vi "MainPr(Calculation)-41.vi"() -> ()   [LabVIEW 2017]
doc: "Main Program for Tracking\nThis VI Represents Front Panel and Control Buttons for Perform Tracking\nPlease, optimize the front panel for your own monitor resolution and needs"
uses:
  <vilib>/vision/Avi.llb/IMAQ AVI2 Refnum.ctl
  <vilib>/vision/NI_Vision_Development_Module.lvlib
  <vilib>/Utility/config.llb/NI_LVConfig.lvlib
panel:
  out "error out":errorcluster
  in  "STOP Program":bool
  in  "Front Panel":T1(tab)
  in  "FrameCtl":u32 max=299
  out "1st Movie (Comparison)":T2(plugin-control)
  out "1st Movie":T2(plugin-control)
  in  "Gamma":sgl format="%.2f"
  in  "Operator G Correction":T3(ring)
  in  "Parameter LoG":sgl format="%.2f"
  in  "Operator LoG":T3(ring)
  in  "1/2 Channels":bool
  in  "Sigma":dbl min=0.1
  in  "FrameCtl2":u32 max=299
  in  "Gray or Binarized?":bool
  out "1st Movie Original":T2(plugin-control)
  out "1st Movie Processed":T2(plugin-control)
  in  "Index for thresholding":i8 min=-4
  in  "Keep Nega-\ntive Values?":bool
  out "Detection Progress":u8(slide) scale=0.0..100.0
  in  "# of Frame":u32 max=299
  in  "Save pics (ex)":bool
  in  "Find ALL objects":bool
  out "Results on 1st Movie":T2(plugin-control)
  out "1st Filtering":T2(plugin-control)
  in  "Try my filters!":bool
  in  "# Erosion":i32=2
  in  "Connectivity":bool=TRUE
  in  "Min  Diam":dbl
  in  "Max  Diam":dbl min=12.0
  in  "Filter Tracks":bool
  out "Tracking progress":u8(slide) scale=0.0..100.0
  in  "Save pictures":bool
  in  "Save movies":bool
  in  "Frame":u32 max=299
  in  "Delete Tracs":bool
  out "1st Filtered":T2(plugin-control)
  in  "dR max":dbl min=1.0
  out "1st Filtering (NN)":T2(plugin-control)
  in  "dR min":dbl min=0.0 max=11.0
  out "Raw #":i32
  out "Saved #":i32
  in  "Tracking Procedure":bool
  in  "Min TRK L":i32 min=2 max=298 step=1
  in  "Closing gaps":i32 min=1 max=298 step=1
  in  "% linearity":i32 min=1 max=100 step=1
  in  "Max angle":dbl min=0.0 max=89.0 step=1.0
  in  "FPS":u32
  in  "FPS Gr":u32
  in  "Save videos \nbelow as *avi":bool
  in  "Save pics below":bool
  in  "Testing Frame":u32 max=17
  out "After Resolving Correspondence Problem":T2(plugin-control)
  out "Connected and Grouped Tracks":T2(plugin-control)
  in  "Tracks group":i32 min=0 max=394
  in  "Save Tracks in Columns (x,y,dx,dy)":bool
  in  "Save Duration of Tracks":bool
  in  "Save Mean Velocities":bool
  out "Duration of Tracks":T4(graph)
  out "Mean Instant Velocities for Each Track":T4(graph)
  in  "Show Distributions":bool
  out "All Path Vels":T4(graph)
  out "All Instant Vels":T4(graph)
  out "mean Instant Vel":dbl format="%#_1f"
  out "StD Instant":dbl format="%#_1g"
  out "mean Path Vel":dbl format="%.1f"
  out "StD Path":dbl format="%.1f"
  in  "Bins":i32=10
  in  "Save All Instant Vels":bool
  in  "Save Path Velocities":bool
  # "Two channels"
  # "*Planning develop-\nment switcher (old)"
  # "One channel"
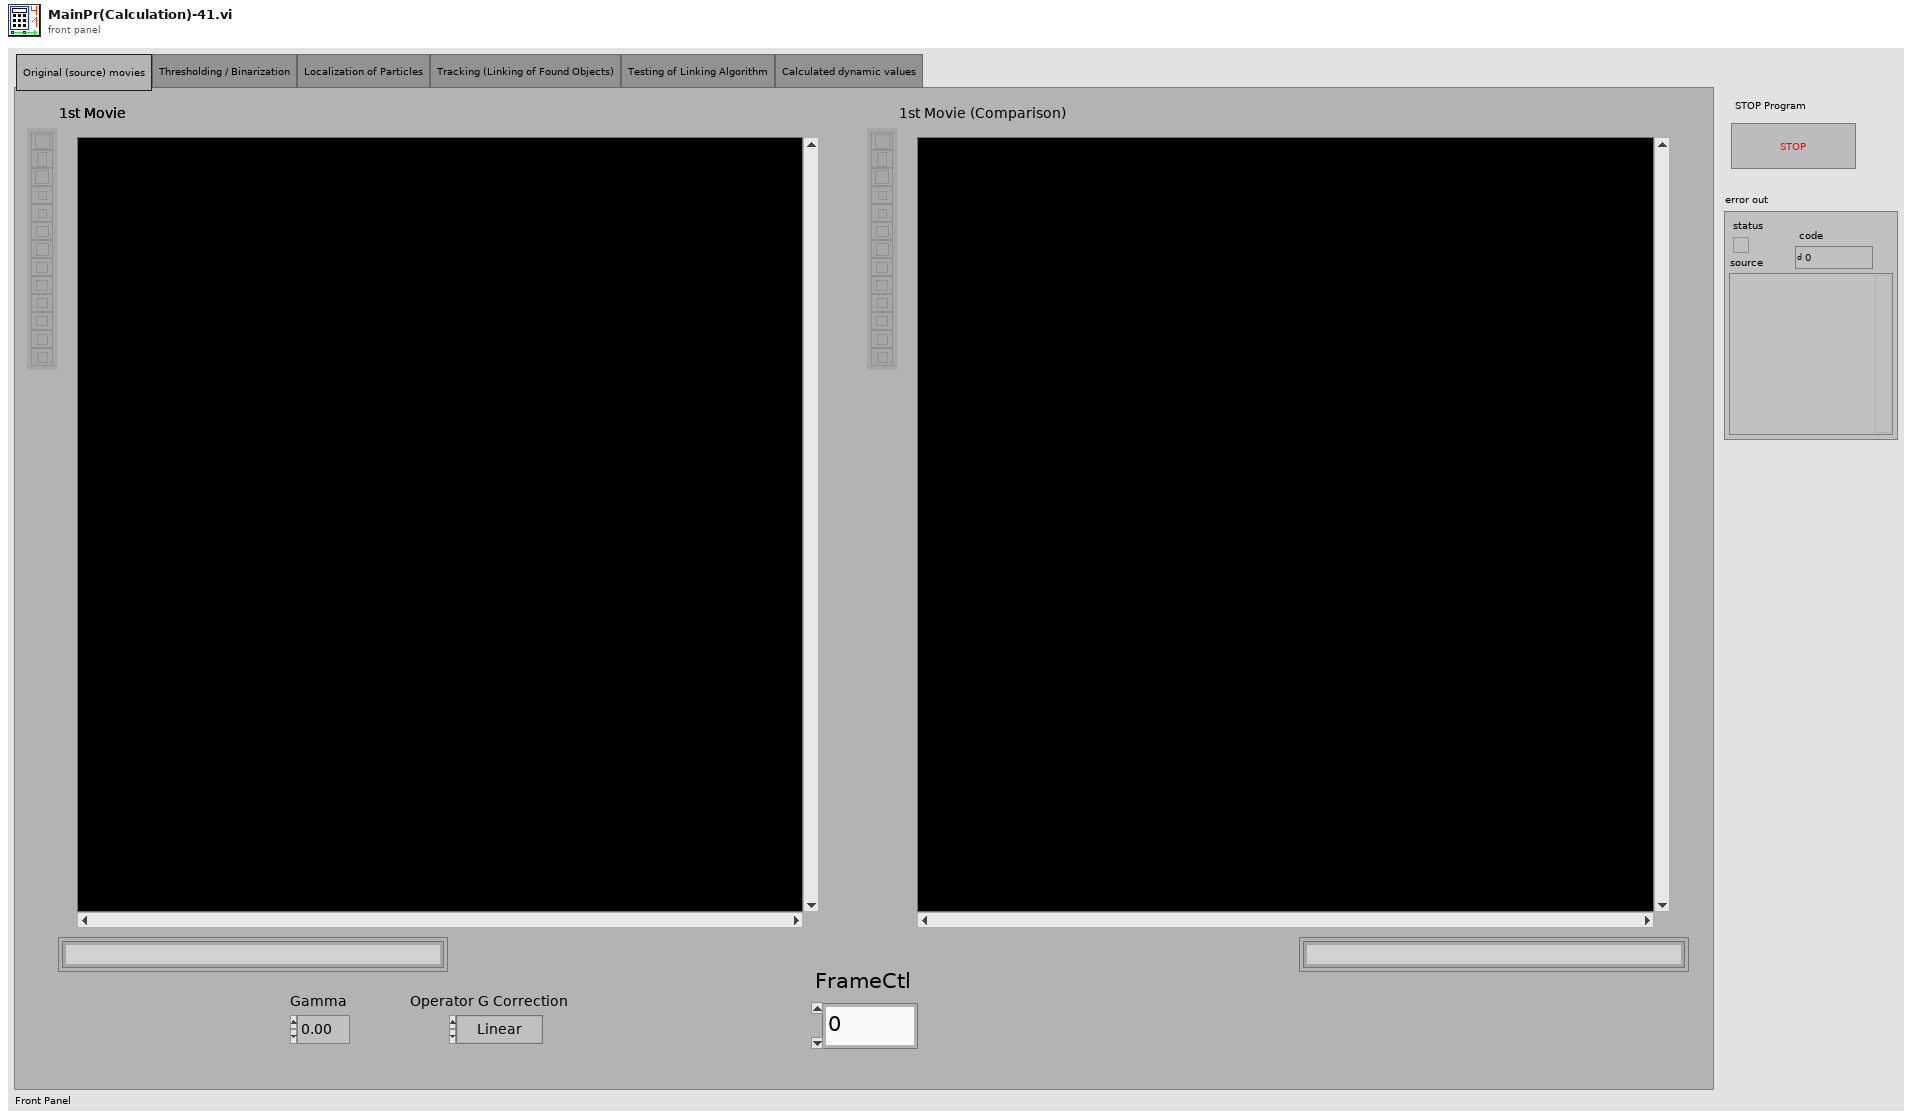
[diagram p1: front panel]
types:
  T1 = enum32{"Original (source) movies", "Thresholding / Binarization", "Localization of Particles", "Tracking (Linking of Found Objects)", "Testing of Linking Algorithm", "Calculated dynamic values"}
  T2 = typedef "IMAQ Image.ctl" = refnum<image>
  T3 = enum32{"Linear", "Log", "Exp", "Square", "Square root", "Power X", "Power 1/X"}
  T4 = cluster{"X Values":dbl[], "Histogram: h(x)":i32[]}
  T5 = typedef "IMAQ AVI2 Refnum.ctl" = refnum<k20>
  T6 = typedef "Image Type" = u32
  T7 = typedef "Particle Parameters" = i32
  T8 = cluster{"[IN] AVI Refnum":T5, "[IN] Image Type":T6, "[IN] Particle Filter Setups":cluster{"Erosion":i32, "Connectivity ":bool, "Type of particle filter":cluster{"Measurement Parameter":T7, "Min  Diam":dbl, "Max  Diam":dbl, "Range":bool, "Range":bool}[]}, "[IN] # Channel":u8, "[IN] Keep Nega-\ntive Values?":bool, "[IN] Image Filtering Settings":cluster{"Gamma Origin":sgl, "Operator Origin":enum32{"Linear", "Log", "Exp", "Square", "Square root", "Power X", "Power 1/X"}, "Gamma LoG":sgl, "Operator LoG":enum32{"Linear", "Log", "Exp", "Square", "Square root", "Power X", "Power 1/X"}, "Sigma":dbl, "Thresholding Index":i8}, "[IN] Binarization Settings":cluster{"MinBin2":sgl, "MaxBin2":sgl}[]}
  T9 = enum8{"Enabled", "Disabled", "Disabled and Grayed Out"}
  T10 = cluster{"dR min ":dbl, "dR max ":dbl, "Closing gaps":i32, "Min TRK L":i32, "% linearity":i32, "Max angle":dbl, "Tracking progress":refnum<vi>}
  T11 = typedef "NI_LVConfig.lvlib/Config Data RefNum.ctl" = refnum<k1>
  T12 = cluster{"X,Y":dbl[][], "Areas particles":dbl[][], "Particle Fil Setups":cluster{"Erosion":i32, "Connectivity ":bool, "Type of particle filter":cluster{"Measurement Parameter":T7, "Min  Diam":dbl, "Max  Diam":dbl, "Range":bool, "Range":bool}[]}, "Tracks, Coordinates":cluster{"(X,Y) Unmoved":dbl[][], "(X,Y,dX,dY) Dur 1 Frame":dbl[][], "(X,Y,dX,dY) W/t Problems":dbl[][], "(X,Y,dX,dY) NN filtered":dbl[][], "(X,Y,dX,dY) TH filtered":dbl[][], "Tracks":cluster{"Tracks":dbl[], "Start Pos":i32}[], "Tracks w/t Problems":cluster{"Tracks":dbl[], "Start Pos":i32}[]}}
  T13 = cluster{"Before Grouped Tracks":cluster{"Tracks":dbl[][], "Start Pos":i32[], "Dot Statuses":i16[][]}[], "After Grouped Tracks":cluster{"Tracks":dbl[][], "Start Pos":i32[], "Dot Statuses":i16[][]}[], "Current\nGroup":i32}
  T14 = cluster{"Gamma Origin":sgl, "Operator Origin":enum32{"Linear", "Log", "Exp", "Square", "Square root", "Power X", "Power 1/X"}, "Gamma LoG":sgl, "Operator LoG":enum32{"Linear", "Log", "Exp", "Square", "Square root", "Power X", "Power 1/X"}, "Sigma":dbl, "Thresholding Index":i8}
  T15 = cluster{"Instant Velocities (All)":dbl[], "Path Velocities (All) ":dbl[], "Tracks in columns":dbl[][], "Mean Instant Velo\ncities for Tracks":dbl[], "MSD":dbl[], "Track duration in frames":u16[], "Track length in pixels":dbl[]}
  T16 = cluster{"Starting Value":sgl, "Incremental Value":sgl, "Histogram":u32[]}
  T17 = cluster{"Erosion":i32, "Connectivity ":bool, "Type of particle filter":cluster{"Measurement Parameter":T7, "Min  Diam":dbl, "Max  Diam":dbl, "Range":bool, "Range":bool}[]}
  T18 = cluster{"Measurement Parameter":T7, "Min  Diam":dbl, "Max  Diam":dbl, "Range":bool, "Range":bool}[]
  T19 = cluster{"Tracks W/T Problems":dbl[], "Start Pos":i32}[]
  T20 = cluster{"All Instant Vel-s":cluster{"X Values":dbl[], "Histogram: h(x)":i32[]}, "mean":dbl, "standard deviation":dbl, "All Path Vel-s":cluster{"X Values":dbl[], "Histogram: h(x)":i32[]}, "mean":dbl, "standard deviation":dbl, "Mean Instan Vel-s":cluster{"X Values":dbl[], "Histogram: h(x)":i32[]}, "mean":dbl, "standard deviation":dbl, "Duration of tracks":cluster{"X Values":dbl[], "Histogram: h(x)":i32[]}, "mean":dbl, "standard deviation":dbl}
  T21 = cluster{"(X,Y) Unmoved":dbl[][], "(X,Y,dX,dY) Dur 1 Frame":dbl[][], "(X,Y,dX,dY) W/t Problems":dbl[][], "(X,Y,dX,dY) NN filtered":dbl[][], "(X,Y,dX,dY) TH filtered":dbl[][], "Tracks":cluster{"Tracks":dbl[], "Start Pos":i32}[], "Tracks w/t Problems":cluster{"Tracks":dbl[], "Start Pos":i32}[]}
  T22 = cluster{"Tracks":dbl[][], "Start Pos":i32[], "Dot Statuses":i16[][]}[]
  T23 = cluster{"[IN] Grouped Tracks":cluster{"Tracks":dbl[][], "Start Pos":i32[], "Dot Statuses":i16[][]}[], "[IN] Tracks group":i32, "[IN] Testing Frame ":u32}
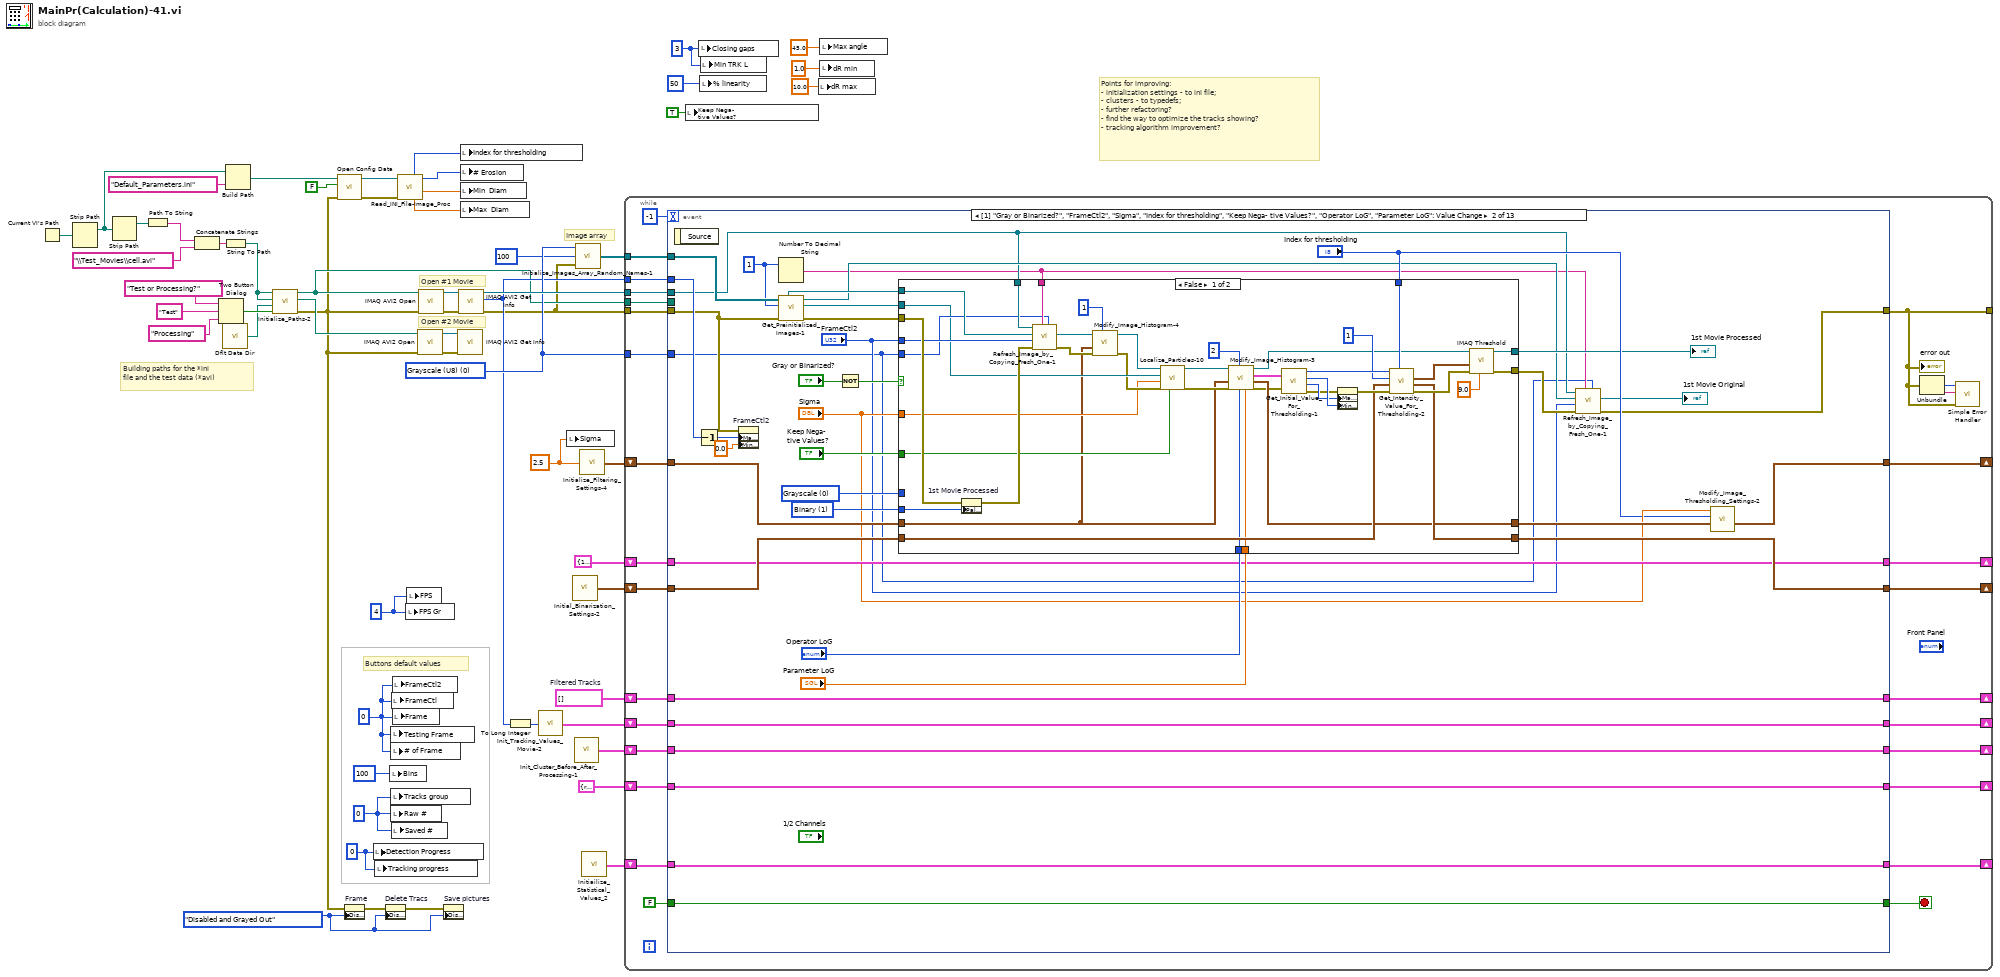
[diagram p0: block diagram]
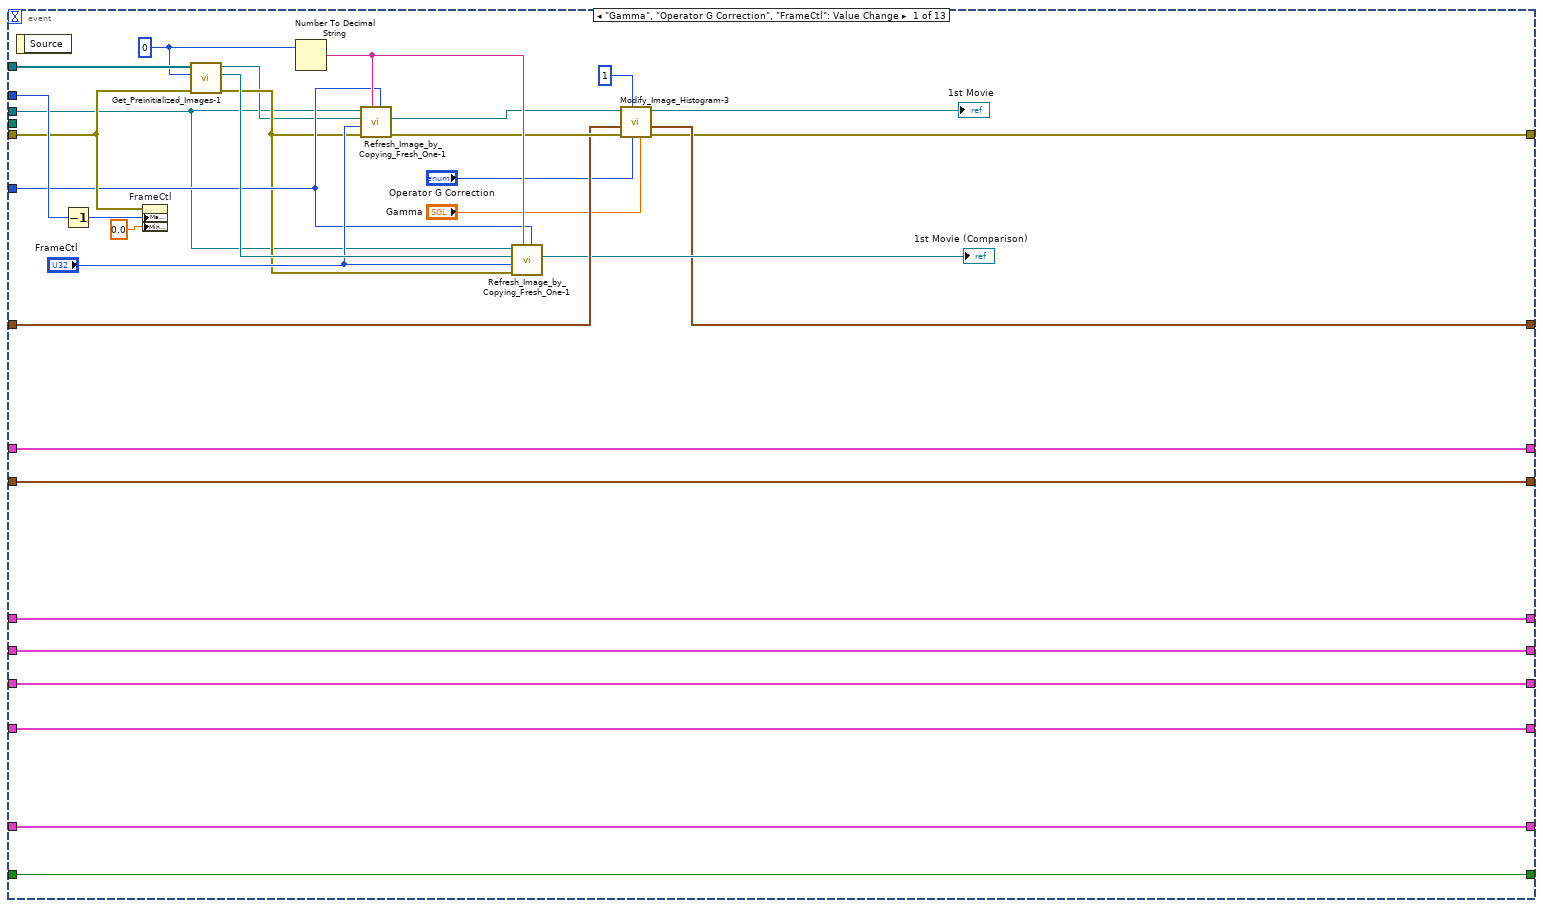
[diagram p2: hidden frame]
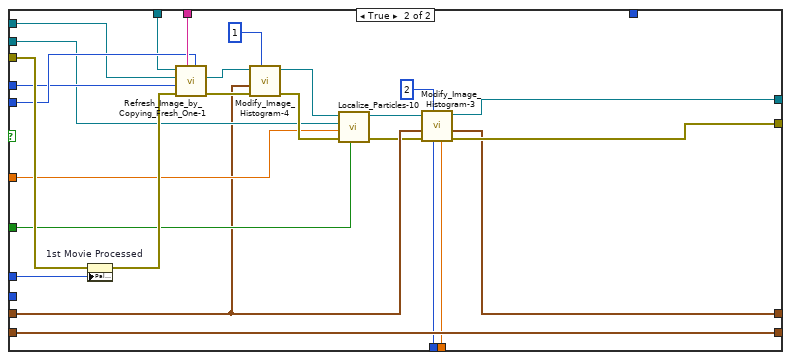
[diagram p3: hidden frame]
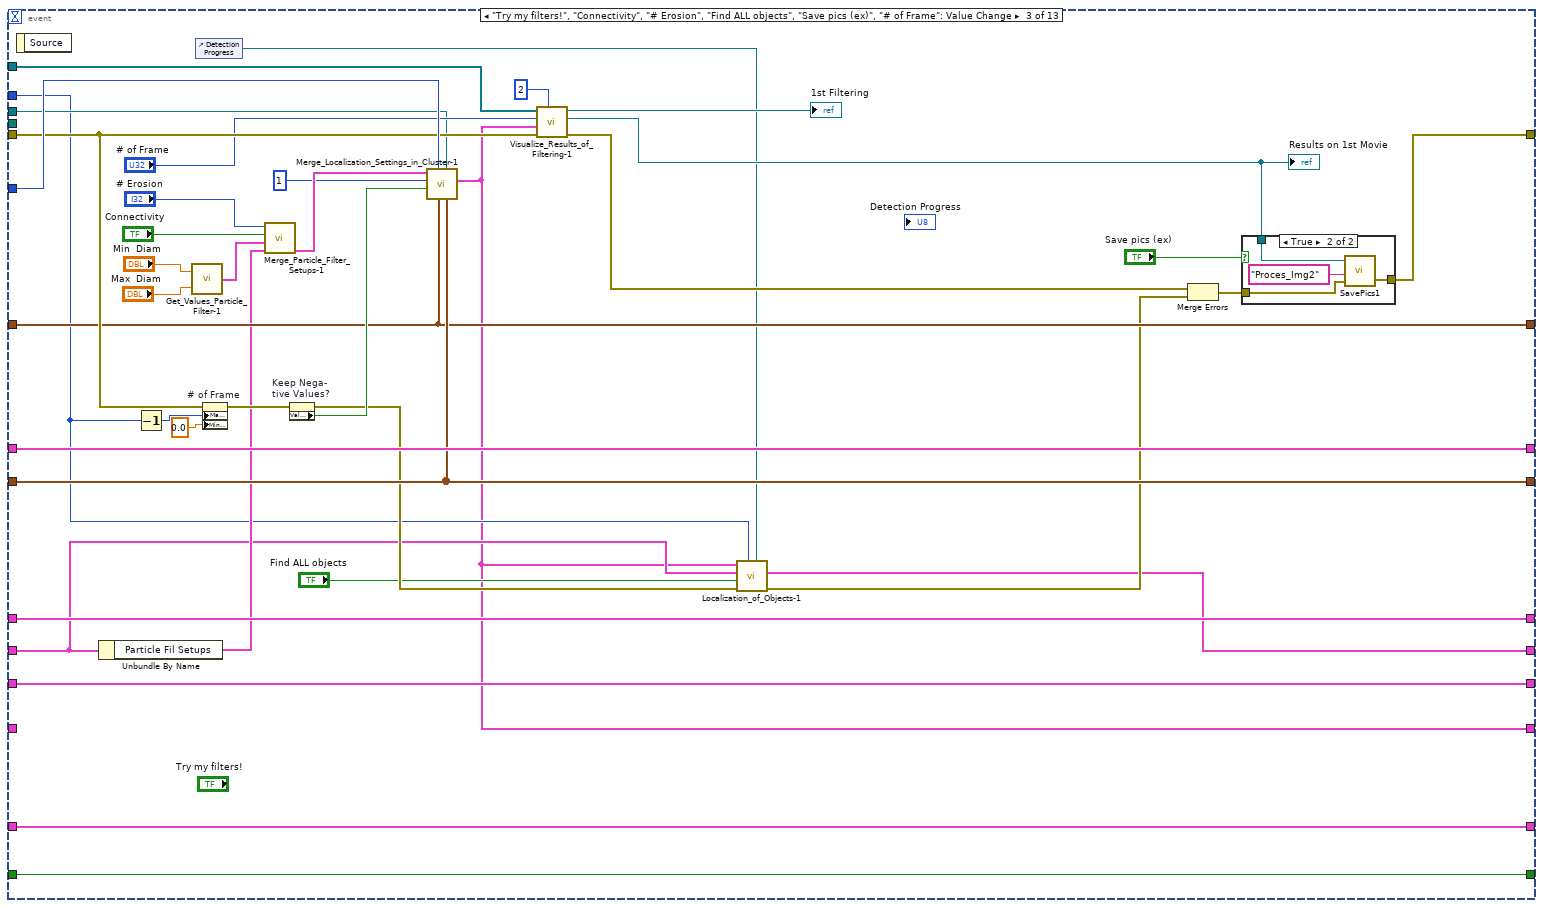
[diagram p4: hidden frame]
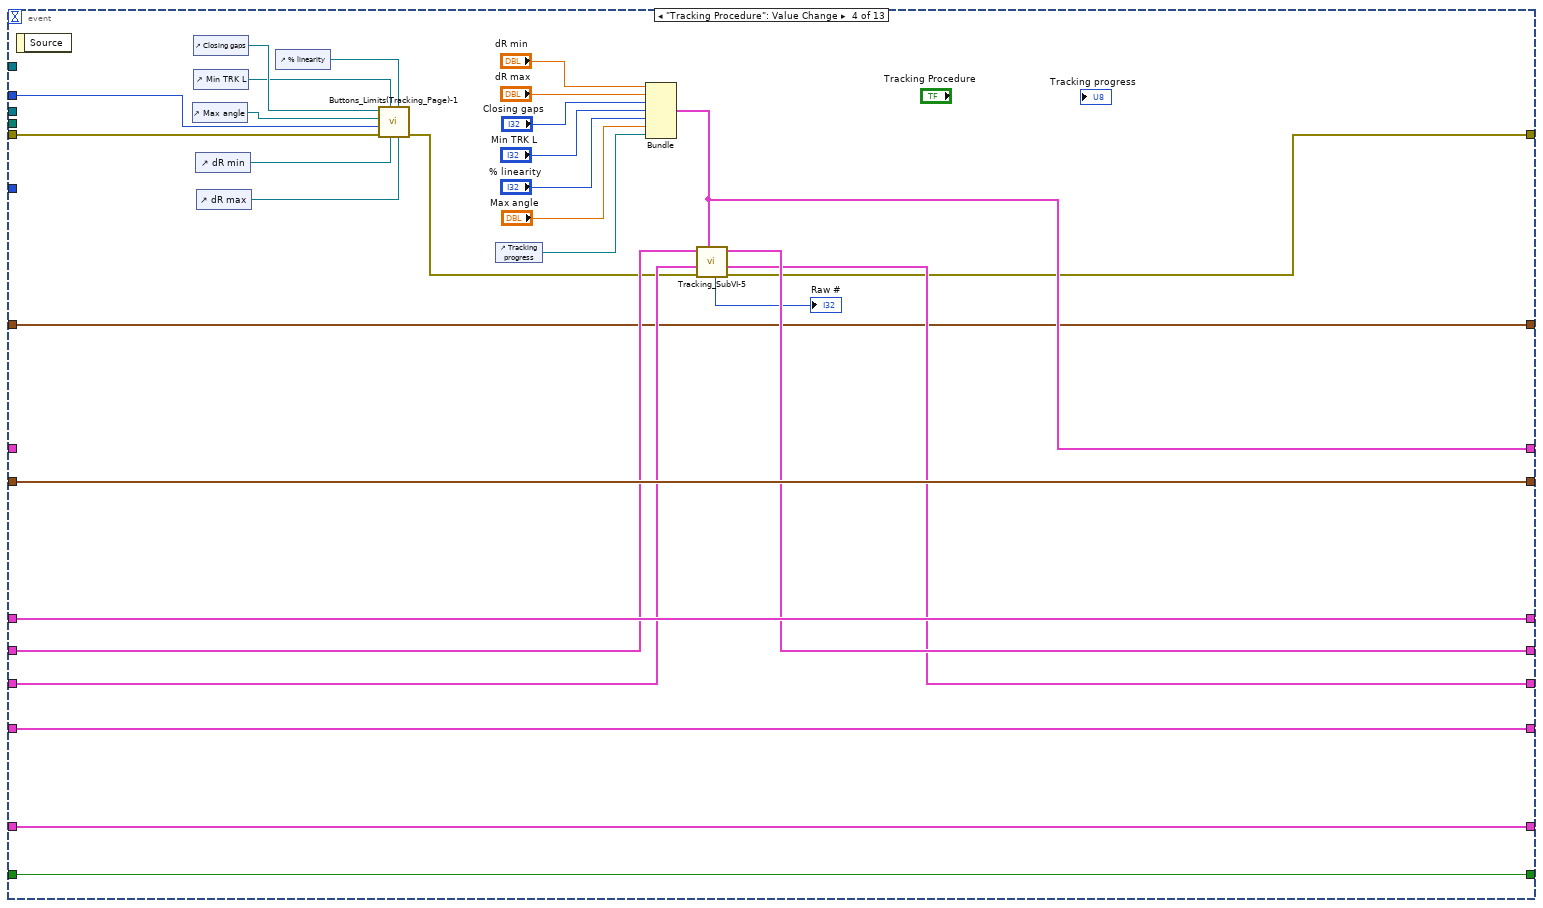
[diagram p6: hidden frame]
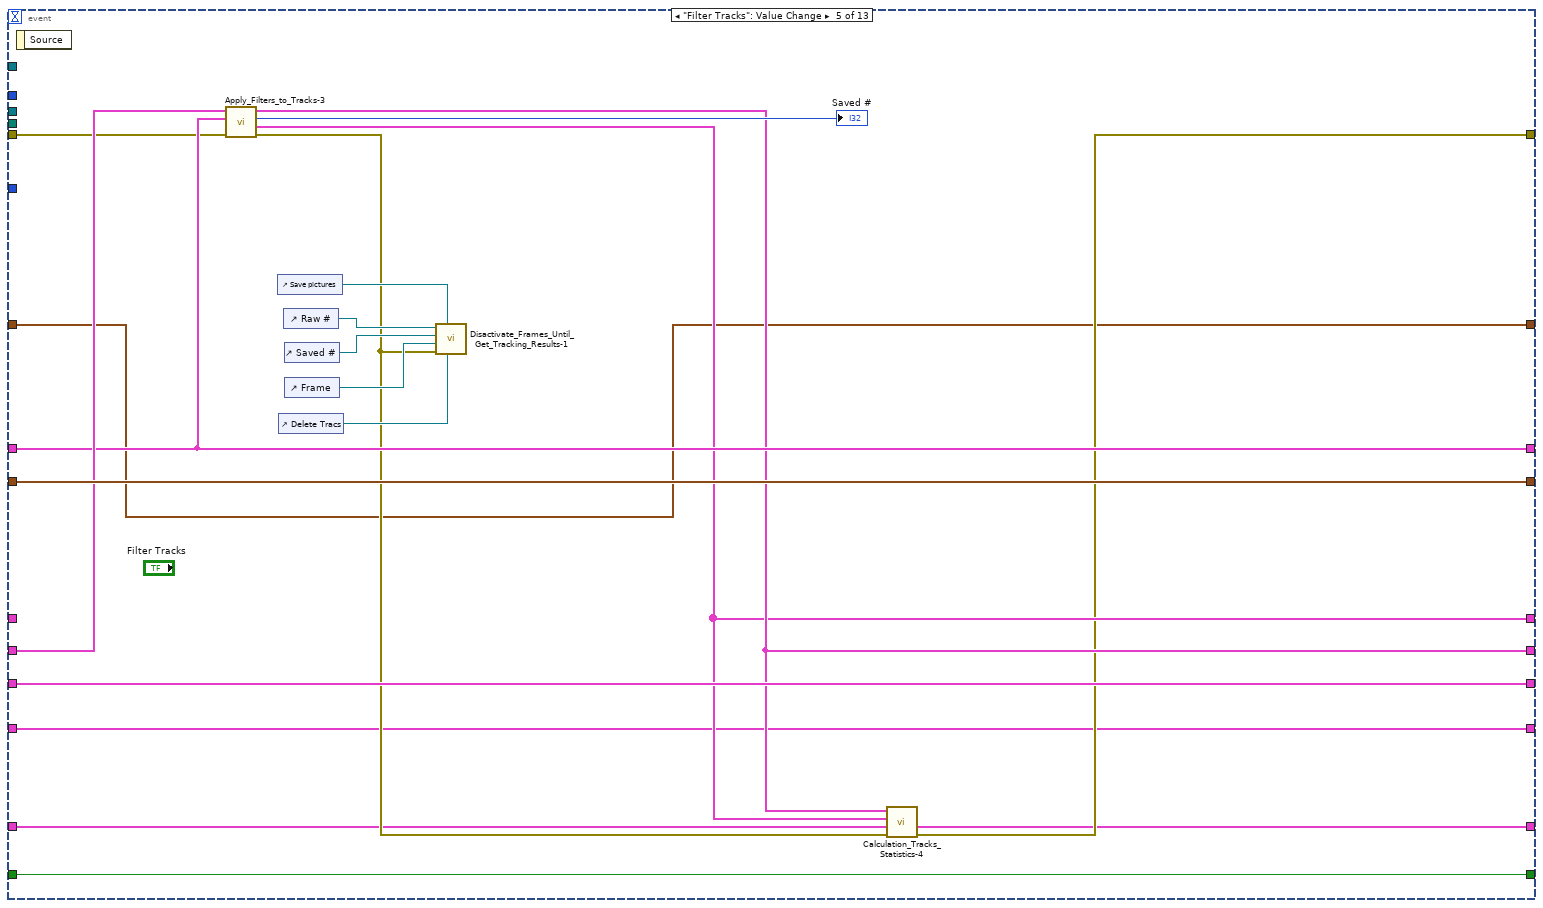
[diagram p7: hidden frame]
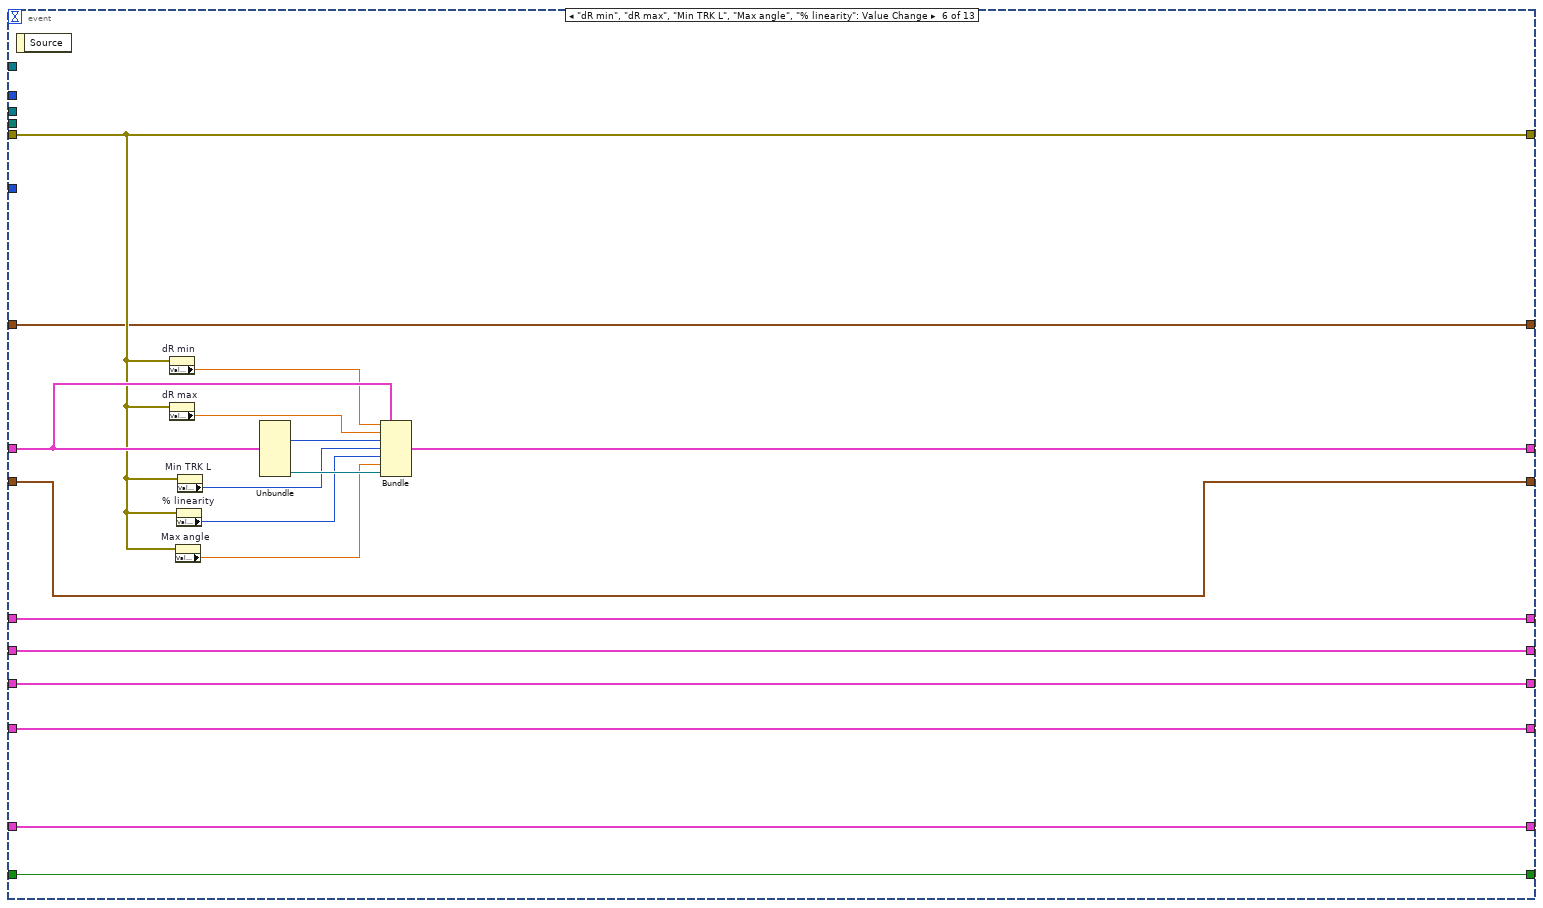
[diagram p8: hidden frame]
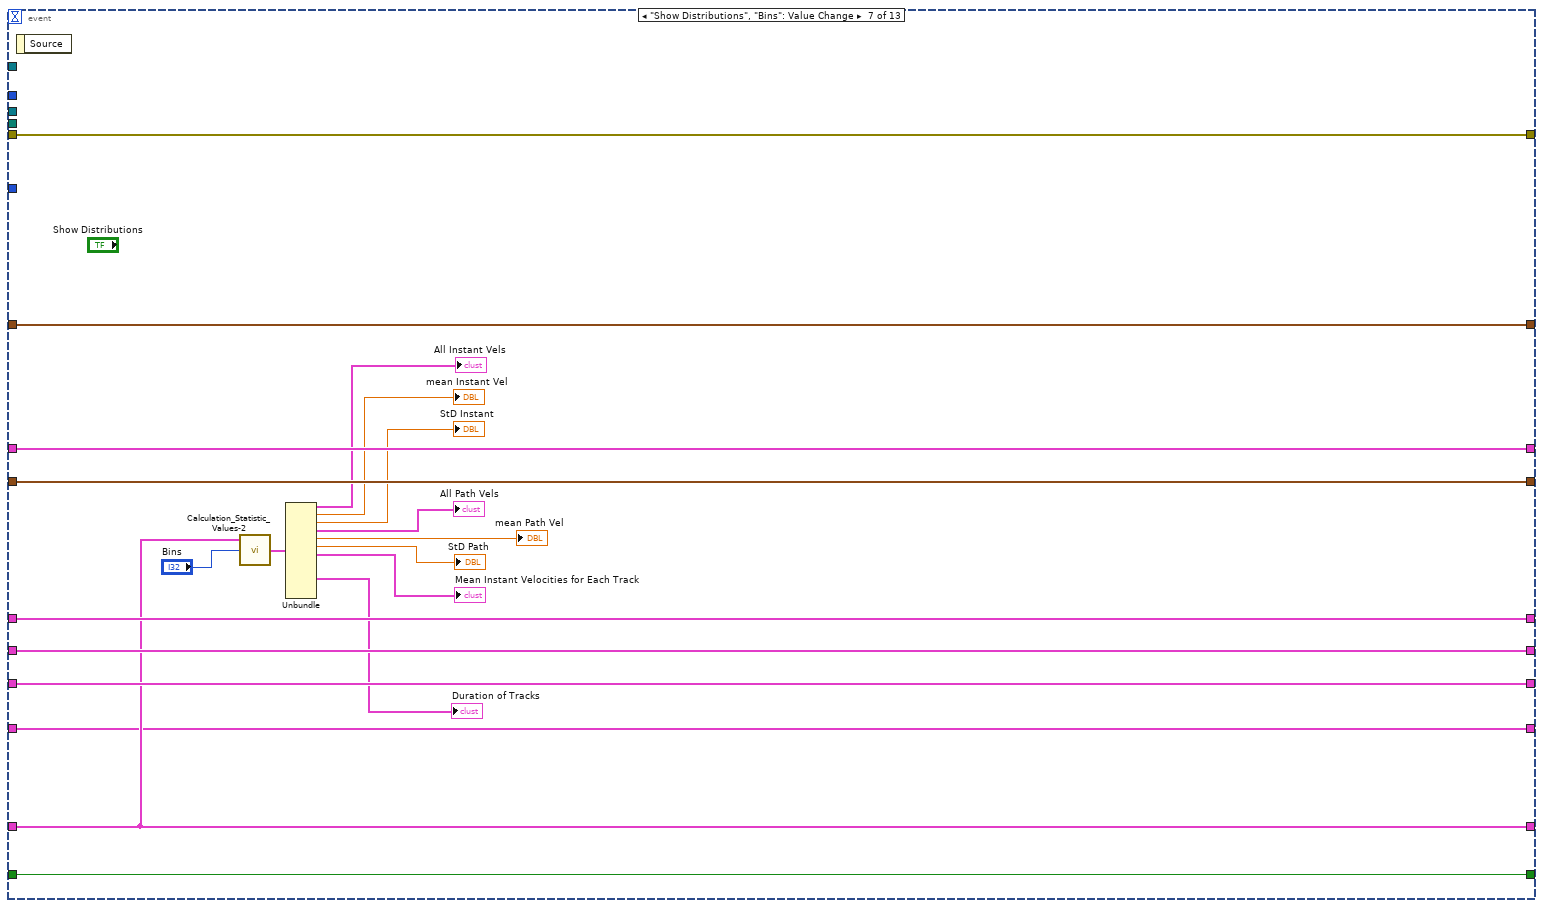
[diagram p9: hidden frame]
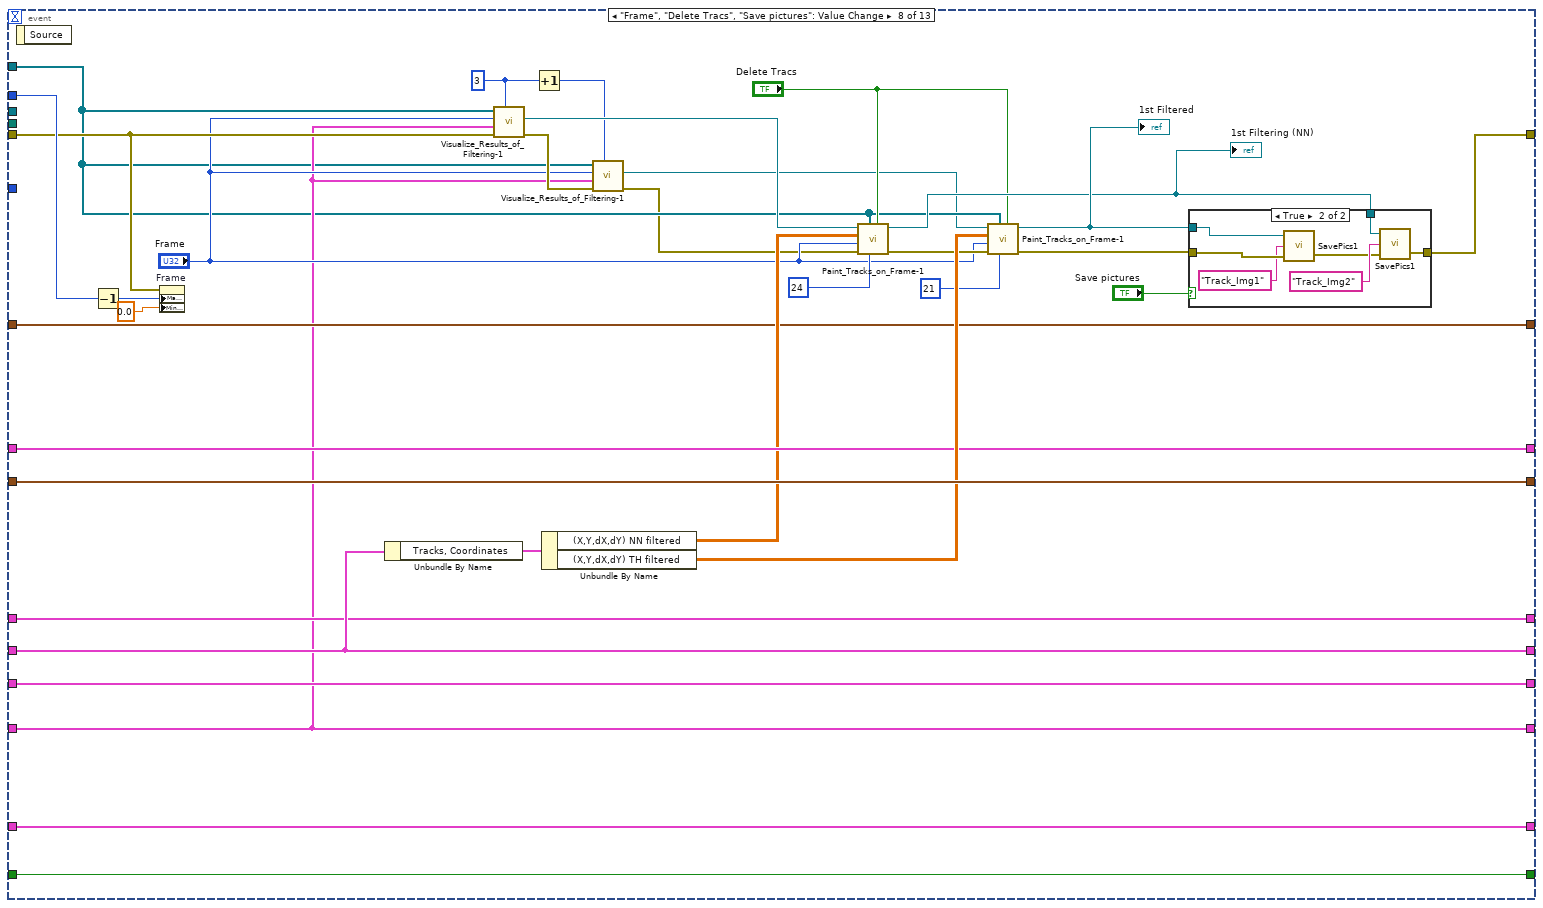
[diagram p10: hidden frame]
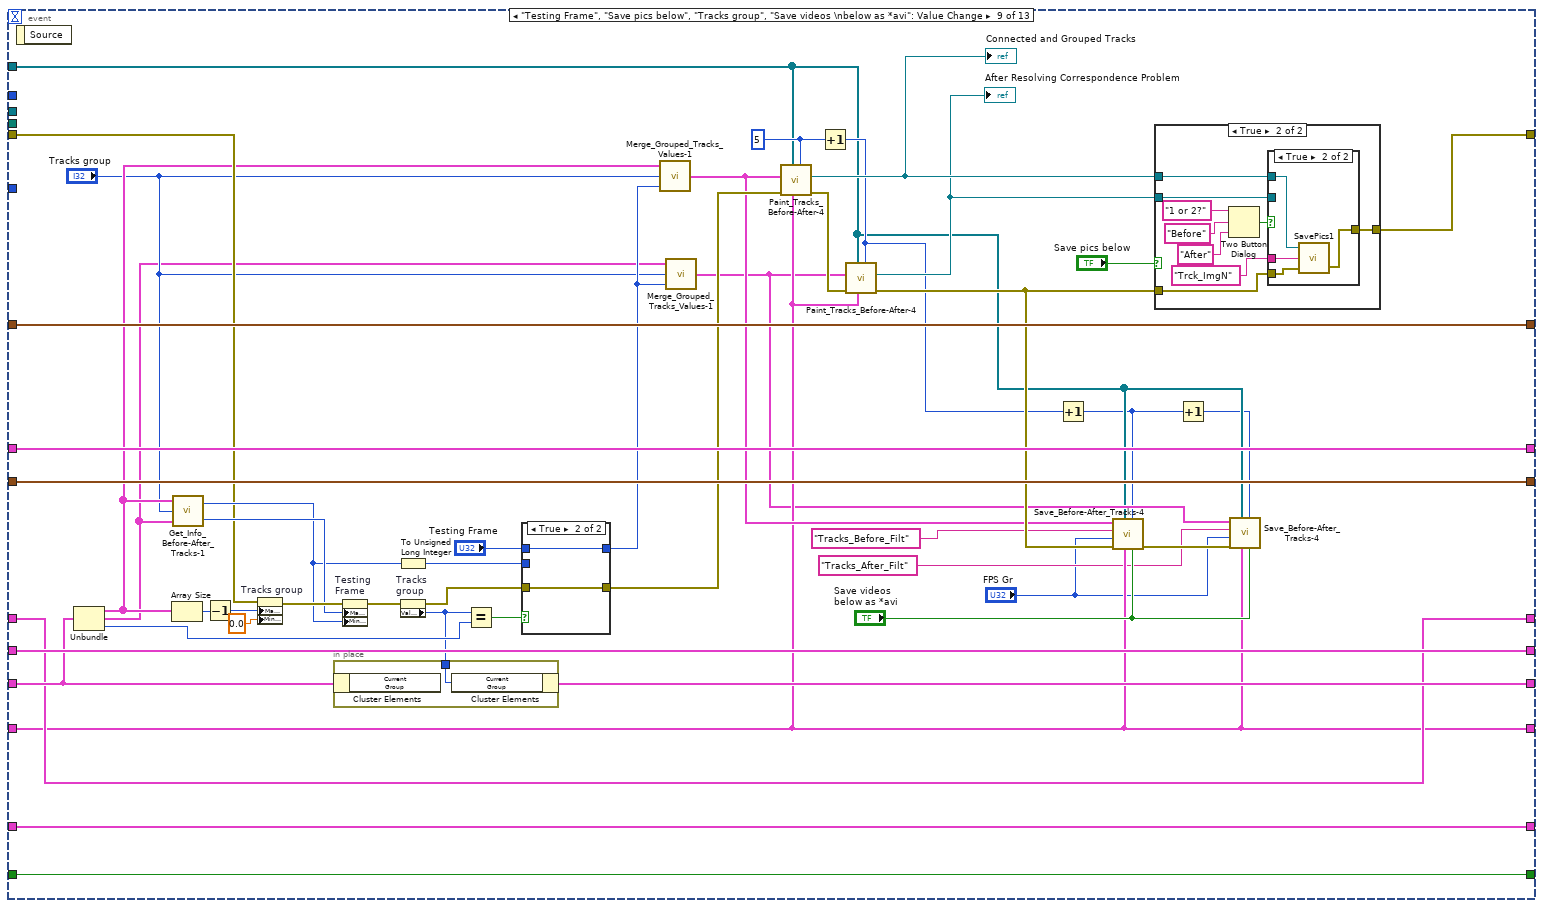
[diagram p12: hidden frame]
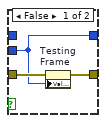
[diagram p13: hidden frame]
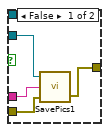
[diagram p15: hidden frame]
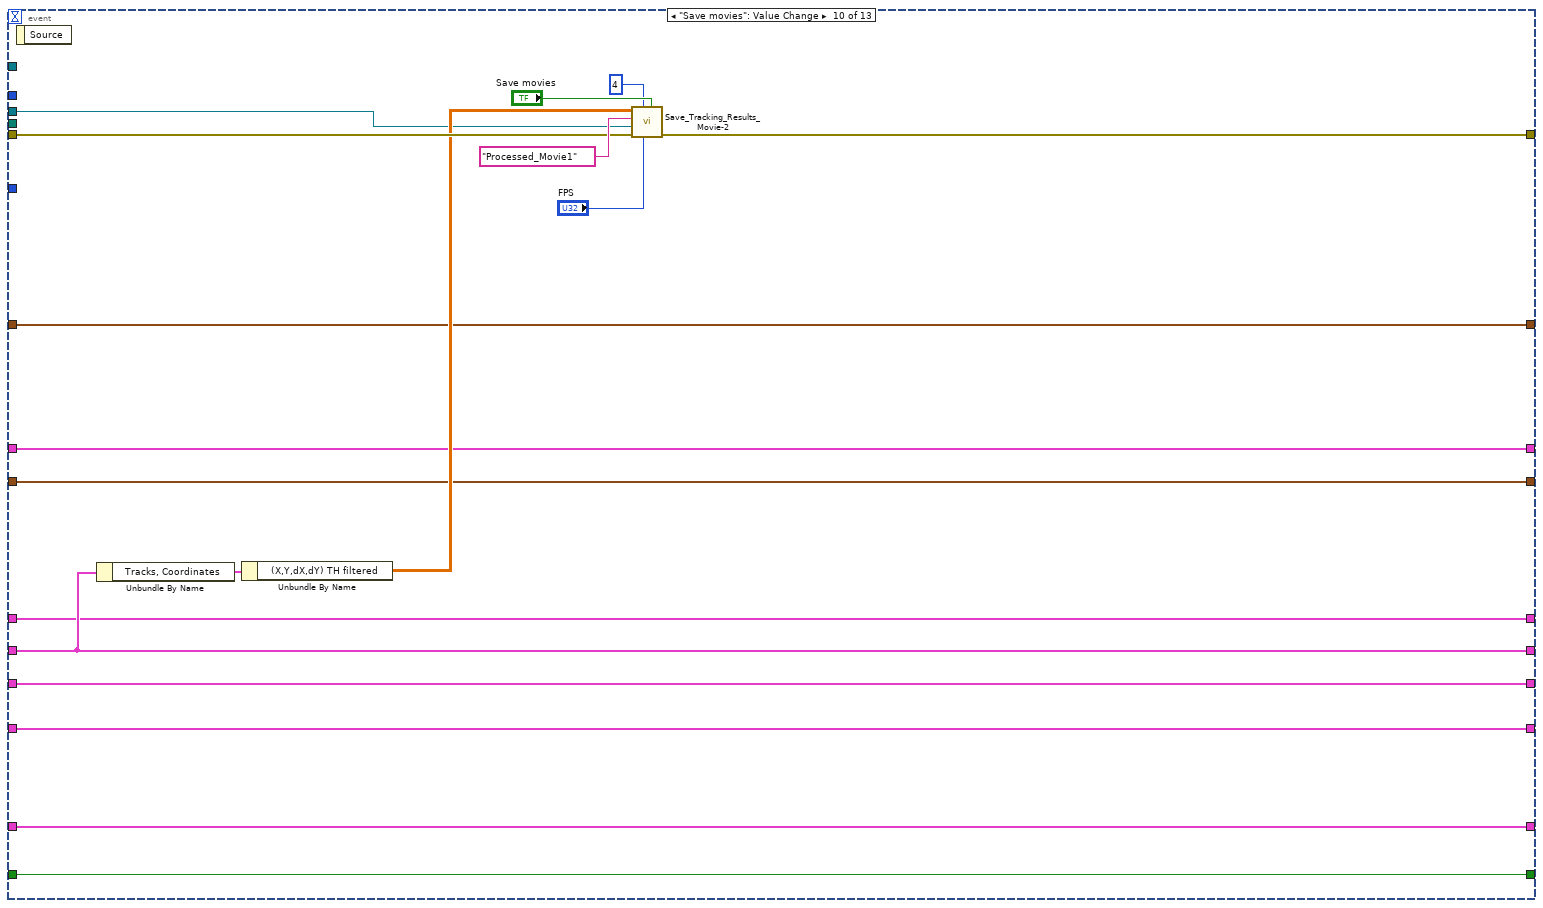
[diagram p16: hidden frame]
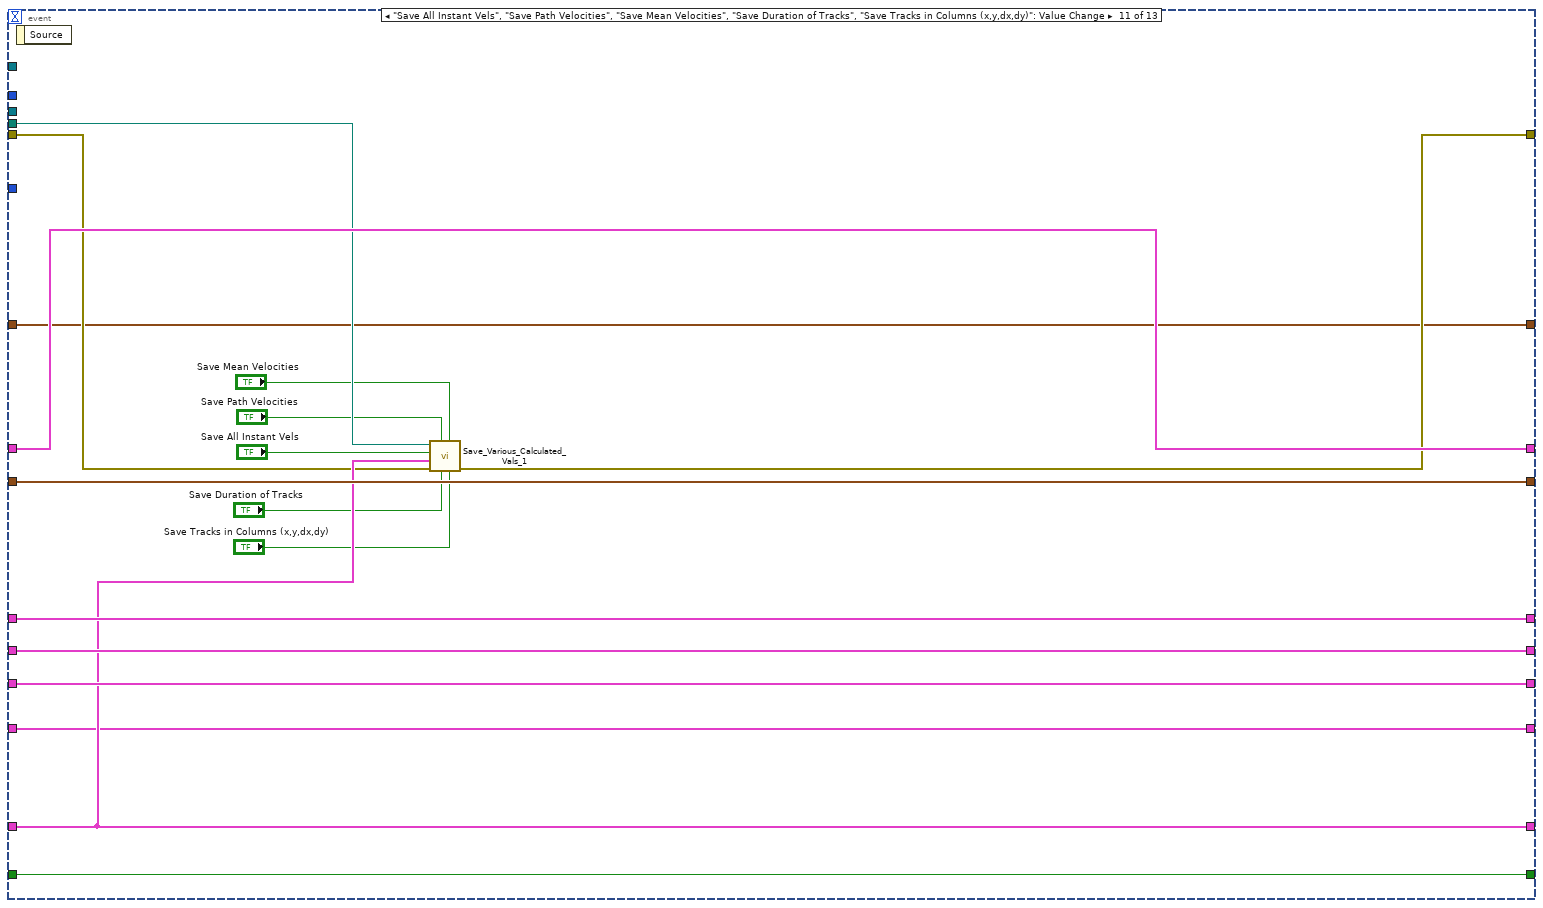
[diagram p17: hidden frame]
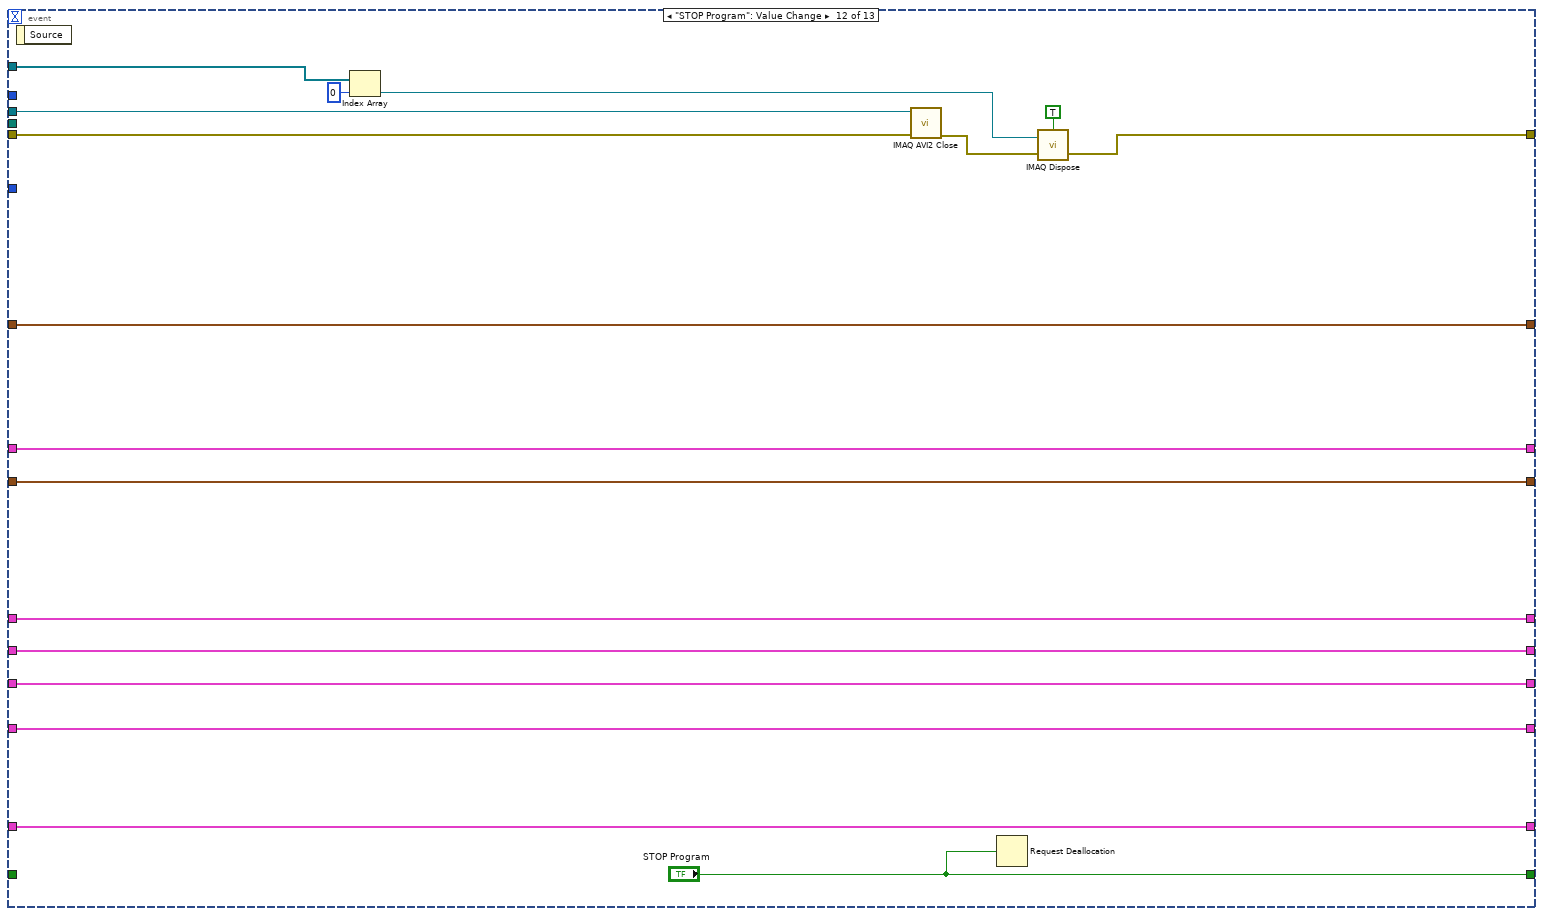
[diagram p18: hidden frame]
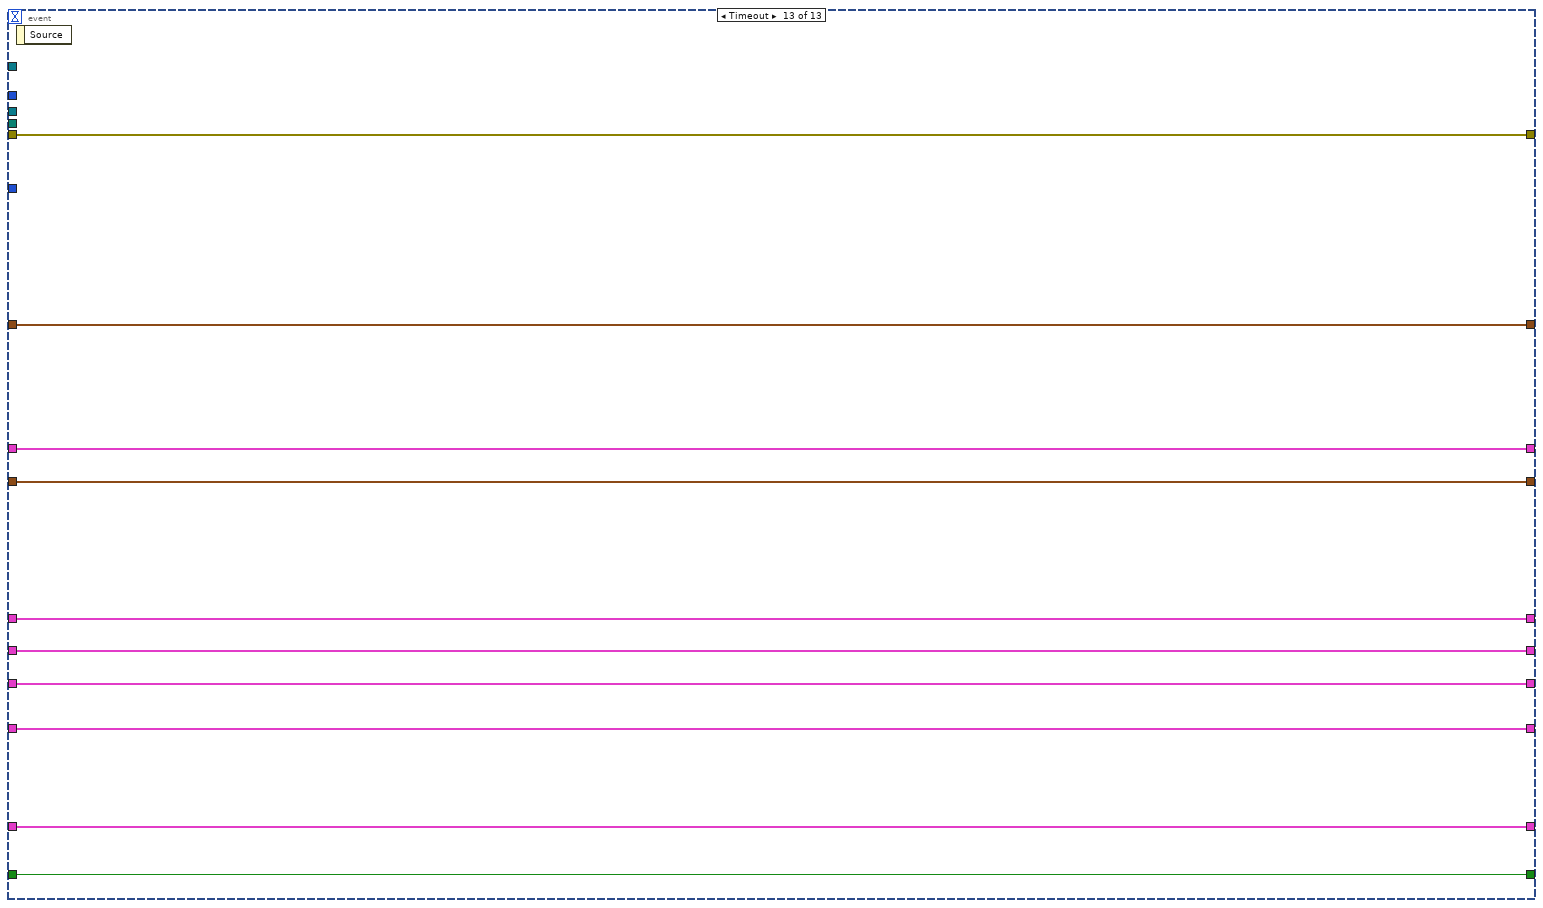
[diagram p19: hidden frame]
diagram:
  w18 = 0 ("Tracks group")
  w19 = u32 4 ("FPS")
  w30 = cluster{"Tracks":dbl[], "Start Pos":i32}[] []  # Filtered Tracks
  w31 = T9."Disabled and Grayed Out" ("Disabled")
  w22 = u32 0 ("Testing Frame")
  w24 = u8 0 ("Progress")
  w25 = 2.5 ("Sigma")
  w17 = 3 ("Closing gaps")
  w49 = T6 0 items=["Grayscale (U8)", "Grayscale (I16)", "Grayscale (SGL)", "Complex (CSG)", "RGB (U32)", "HSL (U32)", "RGB (U64)", "Grayscale (U16)"] ("Image Type")
  # "Buttons default values"
  # "Building paths for the *ini \nfile and the test data (*avi)"
  # "Points for improving:\n- initialization settings - to ini file; \n- clusters - to typedefs; \n- further refactoring?\n- find the way to optimize the tracks showing? \n- tracking algorithm improvement?"
  # "Image array"
  # "Open #2 Movie"
  # "Open #1 Movie"
  n1 = Current VI's Path() -> (path=w11:path)
  n2 = Strip Path(path=w11) -> (stripped path=w7:path)  [unwired: 1 out]
  n3 = Strip Path(path=w7) -> (stripped path=w8:path)  [unwired: 1 out]
  n4 = Path To String(path=w8) -> (string=w42:string)
  n5 = Concatenate Strings(w42, "\\Test_Movies\\cell.avi" ("string")) -> (w39:string)
  n6 = Two Button Dialog(message="Test or Processing?", 1:"Processing" ("F button name (\"Cancel\")"), 2:"Test" ("T button name (\"OK\")")) -> (T button?=w45:bool)
  n7 = call <vilib>:"Dflt Data Dir.vi"() -> ("App:Default Data Directory"=w40:path)
  n8 = String To Path(string=w39) -> (path=w38:path)
  n9 = Build Path(base path=w7, name or relative path="Default_Parameters.ini" ("string")) -> (appended path=w9:path)
  n10 = call "Initialize_Paths-2.vi"("Test or Processing?"=w45, "start path"=w40, "AVI File Path #2"=w38, "AVI File Path #1"=w38) -> ("ERROR OUT"=w12:errorcluster, "AVI File Path #2 OUT"=w44:path, "AVI File Path #1 OUT"=w37:path)  [unwired: 1 out]
  n11 = call <vilib>:"Open Config Data.vi"("error in (no error)"=w12, "create file if necessary (T)"=FALSE, "configuration file path"=w9) -> ("error out"=w5:errorcluster, "refnum"=w6:T11)  [unwired: 6 in, 1 out]
  n12 = property on="Frame" class="DigNum (strict)"(error in=w12, "DisabledEnum"=w31) -> (error out=w33:errorcluster)  [unwired: 1 in, 1 out]
  n13 = local write "Detection Progress"(w24) -> ()
  n14 = local write "Tracking progress"(w24) -> ()
  n15 = property on="Delete Tracs" class="Bool"(error in=w33, "DisabledEnum"=w31) -> (error out=w32:errorcluster)  [unwired: 1 in, 1 out]
  n16 = local write "Bins"(100 ("Intervals")) -> ()
  n17 = local write "Testing Frame"(w22) -> ()
  n18 = local write "# of Frame"(w22) -> ()
  n19 = local write "Tracks group"(w18) -> ()
  n20 = local write "Raw #"(w18) -> ()
  n21 = local write "FrameCtl"(w22) -> ()
  n22 = local write "Saved #"(w18) -> ()
  n23 = local write "FrameCtl2"(w22) -> ()
  n24 = local write "Frame"(w22) -> ()
  n25 = call "Read_INI_File-Image_Proc.vi"("ERROR IN"=w5, "[IN] refnum - ini file"=w6) -> ("[OUT] Minimal diameter"=w3:dbl, "[OUT] Erosion Number"=w2:i32, "[OUT] Maximal diameter"=w1:dbl, "[OUT] Index for thresholding"=w4:i8)  [unwired: 5 in, 1 out]
  n26 = local write "FPS Gr"(w19) -> ()
  n27 = local write "FPS"(w19) -> ()
  n28 = call "IMAQ AVI2 Open"("error in (no error)"=w12, "AVI File Path"=w44) -> ("error out"=w56:errorcluster, "AVI Refnum"=w55:T5)  [unwired: 8 in]
  n29 = call "IMAQ AVI2 Open"("error in (no error)"=w12, "AVI File Path"=w37) -> ("error out"=w57:errorcluster, "AVI Refnum"=w58:T5)  [unwired: 8 in]
  n30 = property on="Save pictures" class="Bool"(error in=w32, "DisabledEnum"=w31) -> ()  [unwired: 1 in, 2 out]
  n31 = call "IMAQ AVI2 Get Info"("error in (no error)"=w56, "AVI Refnum"=w55) -> ()  [unwired: 5 in, 5 out]
  n32 = call "IMAQ AVI2 Get Info"("error in (no error)"=w57, "AVI Refnum"=w58) -> ("error out"=w29:errorcluster, "Number of Frames"=w48:u32, "AVI Refnum (duplicate)"=w54:T5)  [unwired: 5 in, 2 out]
  n33 = local write "Index for thresholding"(w4) -> ()
  n34 = local write "# Erosion"(w2) -> ()
  n35 = local write "Min  Diam"(w3) -> ()
  n36 = local write "Max  Diam"(w1) -> ()
  n37 = To Long Integer(number=w48) -> (32bit integer=w35:i32)
  n38 = call "Init_Tracking_Values_Movie-2.vi"("[IN] # Frames"=w35) -> ("[OUT] Movie Values\n(Empty Cluster)"=w34:T12)
  n39 = local write "Sigma"(w25) -> ()
  n40 = call "Initial_Binarization_Settings-2.vi"() -> ("Binarization Settings"=w50:cluster{"MinBin2":sgl, "MaxBin2":sgl}[])
  n41 = call "Init_Cluster_Before_After_Processing-1.vi"() -> ("[OUT] Before-After"=w43:T13)
  n42 = call "Initialize_Images_Array_Random_Names-1.vi"("error IN"=w29, "# Pics"=100, "Image Type"=w49) -> ("Images Array"=w47:T2[])
  n43 = call "Initialize_Filtering_Settings-4.vi"("Sigma #1"=w25) -> ("[OUT] Image Filtering Settings"=w27:T14)
  n44 = call "Initiailize_Statistical_Values_2.vi"() -> ("Statistics"=w28:T15)
  n45 = while {
    tunnel: w29 -> [w80]
    tunnel: w48 -> [w83]
    tunnel: [w75] -> _
    tunnel: w54 -> [w84]
    shift-right: [w78] -> _
    shift-left: w34 -> [w79]
    shift-right: [w76] -> _
    shift-left: w28 -> [w77]
    shift-right: [w73] -> _
    shift-left: w43 -> [w74]
    shift-right: [w71] -> _
    shift-left: w50 -> [w72]
    tunnel: w49 -> [w70]
    tunnel: w47 -> [w69]
    tunnel: w37 -> [w67]
    shift-right: [w66] -> _
    shift-left: T10 {"dR min "=1.0, "dR max "=10.0, "Closing gaps"=3, "Min TRK L"=3, "% linearity"=50, "Max angle"=46.0, "Tracking progress"=refnum} -> [w65]
    shift-right: [w63] -> _
    shift-left: w30 -> [w64]
    shift-right: [w61] -> _
    shift-left: w27 -> [w62]
    shift-right: [w59] -> _
    shift-left: T8 {"[IN] AVI Refnum"=refnum, "[IN] Image Type"=0, "[IN] Particle Filter Setups"={"Erosion"=0, "Connectivity "=FALSE, "Type of particle filter"=[]}, "[IN] # Channel"=0, "[IN] Keep Nega-\ntive Values?"=FALSE, "[IN] Image Filtering Settings"={"Gamma Origin"=0.0, "Operator Origin"=enum."Linear", "Gamma LoG"=0.0, "Operator LoG"=enum."Linear", "Sigma"=0.0, "Thresholding Index"=0}, "[IN] Binarization Settings"=[]} ("[OUT] Localization Settings") -> [w60]
    stop <- w86 stop-if-true
    n46 = event shown="[1] \"Gray or Binarized?\", \"FrameCtl2\", \"Sigma\", \"Index for thresholding\", \"Keep Nega- tive Values?\", \"Operator LoG\", \"Parameter LoG\": Value Change" {
      selector: _ -> [_ _ _ _ _ _ _ _ _ _ _ _ _]
      dyn-events: _ -> [_ _ _ _ _ _ _ _ _ _ _ _ _]
      timeout: -1 -> [_ _ _ _ _ _ _ _ _ _ _ _ _]
      tunnel: [w100 w136 w251 w279 w310 w327 w349 w372 w424 w472 w497 "STOP Program" w522] -> w86
      tunnel: w84 -> [w101 w122 w233 _ _ _ _ _ _ w476 _ w511 _]
      tunnel: w80 -> [w110 w146 w239 w294 w305 w321 w353 w363 w417 w479 w491 w510 w527]
      tunnel: w83 -> [w111 w147 w228 w293 _ _ _ w378 _ _ _ _ _]
      tunnel: [w88 w125 w257 w269 w300 w321 w353 w385 w434 w473 w492 w506 w527] -> w75
      tunnel: w79 -> [w117 w151 w224 w276 w307 w330 w351 w384 w439 w482 w500 w517 w526]
      tunnel: [w117 w151 w226 w272 w303 w330 w351 w384 w439 w482 w500 w517 w526] -> w78
      tunnel: w77 -> [w114 w152 w259 w277 w299 w328 w346 w381 w441 w483 w493 w515 w525]
      tunnel: [w114 w152 w259 w277 w298 w328 w346 w381 w441 w483 w493 w515 w525] -> w76
      tunnel: w74 -> [w113 w150 w256 w274 w309 w329 w350 w379 w423 w481 w499 w514 w524]
      tunnel: [w113 w150 w256 w270 w309 w329 w350 w379 w421 w481 w499 w514 w524] -> w73
      tunnel: w72 -> [w112 w149 w242 w295 w308 w319 w352 w377 w425 w474 w498 w513 w523]
      tunnel: [w112 w148 w242 w295 w308 w319 w352 w377 w425 w474 w498 w513 w523] -> w71
      tunnel: w70 -> [w104 w120 w241 _ _ _ _ _ _ _ _ _ _]
      tunnel: w69 -> [w109 w145 w238 _ _ _ _ w356 w398 _ _ w512 _]
      tunnel: FALSE ("STOP Program") -> [w100 w136 w251 w279 w310 w327 w349 w372 w424 w472 w497 _ w522]
      tunnel: w67 -> [_ _ _ _ _ _ _ _ _ _ w490 _ _]
      tunnel: [w99 w135 w250 w275 w306 w318 w348 w371 w420 w471 w496 w505 w521] -> w66
      tunnel: w65 -> [w99 w135 w250 _ w306 w333 w348 w371 w420 w471 w496 w505 w521]
      tunnel: w64 -> [w98 w134 w249 w278 _ w331 w347 w370 w419 w470 w495 w504 w520]
      tunnel: [w98 w134 w249 w278 w302 w331 w347 w370 w419 w470 w495 w504 w520] -> w63
      tunnel: w62 -> [w95 w132 w232 w268 w297 w317 w335 w364 w418 w467 w485 w502 w519]
      tunnel: [w89 w119 w232 w268 w297 w317 w335 w364 w418 w467 w485 w502 w519] -> w61
      tunnel: w60 -> [w87 w118 _ w267 w296 w316 w334 w357 w401 w466 w484 w501 w518]
      tunnel: [w87 w118 w223 w267 w296 w316 w334 w357 w401 w466 w484 w501 w518] -> w59
      event "Gamma", "Operator G Correction", "FrameCtl": Value Change {
        w108 = i8 0 ("[IN] Number of event")
        n47 = event-data() -> ()  [unwired: 1 in, 1 out]
        n48 = Decrement(x=w111) -> (x-1=w115:u32)
        n49 = property on="FrameCtl" class="DigNum (strict)"(error in=w110, "Maximum"=w115, "Minimum"=0.0 ("Data Entry Limits:Minimum")) -> ()  [unwired: 1 in, 2 out]
        n50 = call "Get_Preinitialized_Images-1.vi"("error IN"=w110, "[IN] Number of event"=w108, "[IN] Images Array"=w109) -> ("error OUT"=w103:errorcluster, "[OUT] Processed Image #1"=w107:T2, "[OUT] Source Image #2"=w102:T2)  [unwired: 1 in, 2 out]
        n51 = Number To Decimal String(number=w108) -> (decimal integer string=w105:string)  [unwired: 1 in]
        n52 = call "Refresh_Image_by_Copying_Fresh_One-1.vi"("[IN] Image Type"=w104, "[IN] Unique ID\n(# of Event)"=w105, "error IN"=w103, "Frame Number"="FrameCtl", "[IN] Preinitialized Image"=w102, "[IN] AVI Refnum"=w101) -> ("error OUT"=w96:errorcluster, "[OUT] Frame"=w97:T2)  [unwired: 1 in, 1 out]
        n53 = call "Refresh_Image_by_Copying_Fresh_One-1.vi"("[IN] Image Type"=w104, "[IN] Unique ID\n(# of Event)"=w105, "error IN"=w103, "Frame Number"="FrameCtl", "[IN] Preinitialized Image"=w107, "[IN] AVI Refnum"=w101) -> ("[OUT] Frame"=→"1st Movie (Comparison)":T2)  [unwired: 1 in, 2 out]
        n54 = call "Modify_Image_Histogram-3.vi"("[IN] Parameter"="Gamma", "[IN] Operator"="Operator G Correction", "1 - Origin\n2 - LoG"=u8 1 ("# channel"), "error IN"=w96, "[IN] Image Filtering Settings"=w95, "[IN] LoG Processed Image"=w97) -> ("error OUT"=w88:errorcluster, "[OUT] Image Filtering Settings"=w89:T14, "[OUT] Histogram Modified Image"=→"1st Movie":T2)  [unwired: 2 in, 1 out]
      }
      event "Gray or Binarized?", "FrameCtl2", "Sigma", "Index for thresholding", "Keep Nega-\ntive Values?", "Operator LoG", "Parameter LoG": Value Change {
        w133 = u32 0 items=["Grayscale", "Binary", "Gradient", "Rainbow", "Temperature", "User Defined"] ("Palette:Palette Type")
        w137 = u32 1 items=["Grayscale", "Binary", "Gradient", "Rainbow", "Temperature", "User Defined"] ("Palette:Palette Type")
        w143 = i8 1 ("[IN] Number of event")
        n55 = event-data() -> ()  [unwired: 1 in, 1 out]
        n56 = Decrement(x=w147) -> (x-1=w153:u32)
        n57 = property on="FrameCtl2" class="DigNum (strict)"(error in=w146, "Maximum"=w153, "Minimum"=0.0 ("Data Entry Limits:Minimum")) -> ()  [unwired: 1 in, 2 out]
        n58 = Number To Decimal String(number=w143) -> (decimal integer string=w121:string)  [unwired: 1 in]
        n59 = call "Get_Preinitialized_Images-1.vi"("error IN"=w146, "[IN] Number of event"=w143, "[IN] Images Array"=w145) -> ("error OUT"=w144:errorcluster, "[OUT] Processed Image #1"=w141:T2, "[OUT] Source Image #2"=w124:T2, "[OUT] Source Image #1"=w142:T2)  [unwired: 1 in, 1 out]
        n60 = Not(x="Gray or Binarized?") -> (.not. x?=w155:bool)
        n61 = case shown="False" w155 {
          tunnel: w144 -> [w196 w222]
          tunnel: [w191 w201] -> w127
          tunnel: [w195 w202] -> w128
          tunnel: "Sigma" -> [w169 w206]
          tunnel: "FrameCtl2" -> [w187 w216]
          tunnel: "Index for thresholding" -> [w182 _]
          tunnel: w149 -> [w180 w221]
          tunnel: [w177 w221] -> w148
          tunnel: w122 -> [w186 w215]
          tunnel: w120 -> [w176 w218]
          tunnel: w121 -> [w189 w220]
          tunnel: w142 -> [w188 w217]
          tunnel: w141 -> [w171 w205]
          tunnel: "Keep Nega-\ntive Values?" -> [w168 w208]
          tunnel: "Parameter LoG" -> [w157 w197]
          tunnel: "Operator LoG" -> [w158 w198]
          tunnel: w137 -> [w184 _]
          tunnel: w133 -> [_ w214]
          tunnel: w132 -> [w163 w203]
          tunnel: [w162 w199] -> w131
          frame False {
            n62 = property on="1st Movie Processed" class="ImageControl"(error in=w196, "Palette Type"=w184) -> (error out=w190:errorcluster)  [unwired: 1 in, 1 out]
            n63 = call "Refresh_Image_by_Copying_Fresh_One-1.vi"("[IN] Image Type"=w176, "[IN] Unique ID\n(# of Event)"=w189, "error IN"=w190, "Frame Number"=w187, "[IN] Preinitialized Image"=w188, "[IN] AVI Refnum"=w186) -> ("error OUT"=w173:errorcluster, "[OUT] Frame"=w175:T2)  [unwired: 1 in, 1 out]
            n64 = call "Modify_Image_Histogram-4.vi"("1 - Origin\n2 - LoG"=u8 1 ("# channel"), "error IN"=w173, "[IN] Image Filtering Settings"=w163, "[IN] LoG Processed Image"=w175) -> ("error OUT"=w170:errorcluster, "[OUT] Histogram Modified Image"=w172:T2)  [unwired: 5 in, 1 out]
            n65 = call "Localize_Particles-10.vi"("Keep Nega-\ntive Values?"=w168, "error IN"=w170, "[IN] Sigma"=w169, "[IN] Destination Image"=w171, "[IN] Frame"=w172) -> ("error OUT"=w164:errorcluster, "[OUT] LoG Processed Image"=w167:T2)  [unwired: 3 in, 1 out]
            n66 = call "Modify_Image_Histogram-3.vi"("[IN] Parameter"=w157, "[IN] Operator"=w158, "1 - Origin\n2 - LoG"=u8 2 ("1 - Origin\n2 - LoG"), "error IN"=w164, "[IN] Image Filtering Settings"=w163, "[IN] LoG Processed Image"=w167) -> ("error OUT"=w161:errorcluster, "[OUT] Image Filtering Settings"=w162:T14, "[OUT] Histogram"=w160:T16, "[OUT] Histogram Modified Image"=w159:T2)  [unwired: 2 in]
            n67 = call "Get_Initial_Value_For_Thresholding-1.vi"("[IN] Histogram Graph"=w160, "error IN"=w161) -> ("[OUT] Index of starting \npoint for thresholding"=w183:i32, "[OUT] Minimal index for \nthresholding (negative)"=w194:i32, "[OUT] Maximal index \nfor thresholding"=w193:i32, "error OUT"=w185:errorcluster)
            n68 = property on="Index for thresholding" class="DigNum (strict)"(error in=w185, "Maximum"=w193, "Minimum"=w194) -> (error out=w181:errorcluster)  [unwired: 1 in, 1 out]
            n69 = call "Get_Intensity_Value_For_Thresholding-2.vi"("[IN] Index for \nthresholding"=w182, "error IN"=w181, "[IN] Binarization Set\ntings (Both Channels)"=w180, "[IN] 1 or 2 channel"=u8 1, "[IN] Index of starting \npoint for thresholding"=w183) -> ("error OUT"=w178:errorcluster, "[OUT] Binarization Set\ntings (Both Channels)"=w177:cluster{"MinBin2":sgl, "MaxBin2":sgl}[], "[OUT] For Operator \nBinarization Values"=w179:cluster{"MinBin2":sgl, "MaxBin2":sgl})  [unwired: 1 in]
            n70 = call "IMAQ Threshold"("Replace Value"=sgl 9.0, "error in (no error)"=w178, "Range"=w179, "Image Src"=w159) -> ("error out"=w191:errorcluster, "Image Dst Out"=w195:T2)  [unwired: 6 in]
          }
          frame True {
            n71 = property on="1st Movie Processed" class="ImageControl"(error in=w222, "Palette Type"=w214) -> (error out=w219:errorcluster)  [unwired: 1 in, 1 out]
            n72 = call "Refresh_Image_by_Copying_Fresh_One-1.vi"("[IN] Image Type"=w218, "[IN] Unique ID\n(# of Event)"=w220, "error IN"=w219, "Frame Number"=w216, "[IN] Preinitialized Image"=w217, "[IN] AVI Refnum"=w215) -> ("error OUT"=w213:errorcluster, "[OUT] Frame"=w212:T2)  [unwired: 1 in, 1 out]
            n73 = call "Modify_Image_Histogram-4.vi"("1 - Origin\n2 - LoG"=u8 1 ("# channel"), "error IN"=w213, "[IN] Image Filtering Settings"=w203, "[IN] LoG Processed Image"=w212) -> ("error OUT"=w207:errorcluster, "[OUT] Histogram Modified Image"=w209:T2)  [unwired: 5 in, 1 out]
            n74 = call "Localize_Particles-10.vi"("Keep Nega-\ntive Values?"=w208, "error IN"=w207, "[IN] Sigma"=w206, "[IN] Destination Image"=w205, "[IN] Frame"=w209) -> ("error OUT"=w200:errorcluster, "[OUT] LoG Processed Image"=w204:T2)  [unwired: 3 in, 1 out]
            n75 = call "Modify_Image_Histogram-3.vi"("[IN] Parameter"=w197, "[IN] Operator"=w198, "1 - Origin\n2 - LoG"=u8 2 ("# channel"), "error IN"=w200, "[IN] Image Filtering Settings"=w203, "[IN] LoG Processed Image"=w204) -> ("error OUT"=w201:errorcluster, "[OUT] Image Filtering Settings"=w199:T14, "[OUT] Histogram Modified Image"=w202:T2)  [unwired: 2 in, 1 out]
          }
        }
        "1st Movie Processed" <- w128
        n76 = call "Refresh_Image_by_Copying_Fresh_One-1.vi"("[IN] Image Type"=w120, "[IN] Unique ID\n(# of Event)"=w121, "error IN"=w127, "Frame Number"="FrameCtl2", "[IN] Preinitialized Image"=w124, "[IN] AVI Refnum"=w122) -> ("error OUT"=w125:errorcluster, "[OUT] Frame"=→"1st Movie Original":T2)  [unwired: 1 in, 1 out]
        n77 = call "Modify_Image_Thresholding_Settings-2.vi"("[IN] Image Filtering Settings"=w131, "[IN] Index for thresholding"="Index for thresholding", "[IN] Sigma"="Sigma") -> ("[OUT] Image Filtering Settings"=w119:T14)  [unwired: 6 in]
      }
      event "Try my filters!", "Connectivity", "# Erosion", "Find ALL objects", "Save pics (ex)", "# of Frame": Value Change {
        n78 = event-data() -> ()  [unwired: 1 in, 1 out]
        n79 = Unbundle By Name(w224) -> ("Particle Fil Setups"=w229:T17)
        n80 = Decrement(x=w228) -> (x-1=w260:u32)
        n81 = call "Get_Values_Particle_Filter-1.vi"("Max  Diam"="Max  Diam", "Min  Diam"="Min  Diam") -> ("type of filters\nparticles search"=w246:T18)
        n82 = control-ref of="Detection Progress"() -> (w230:refnum<vi>)
        n83 = property on="# of Frame" class="DigNum (strict)"(error in=w239, "Maximum"=w260, "Minimum"=0.0 ("Data Entry Limits:Minimum")) -> (error out=w252:errorcluster)  [unwired: 1 in, 1 out]
        n84 = call "Merge_Particle_Filter_Setups-1.vi"("[IN] Particle Filter Setups"=w229, "type of filters\nparticles search"=w246, "Connectivity"="Connectivity", "# Erosion"="# Erosion") -> ("[OUT] Particle Filter Setups"=w245:T17)  [unwired: 3 in]
        n85 = property on="Keep Nega-\ntive Values?" class="Bool (strict)"(error in=w252) -> (error out=w231:errorcluster, "Value"=w243:bool)  [unwired: 1 in, 1 out]
        n86 = call "Merge_Localization_Settings_in_Cluster-1.vi"("[IN] Binarization Settings"=w242, "[IN] AVI Refnum"=w233, "[IN] Image Filtering Settings"=w232, "[IN] Image Type"=w241, "[IN] Keep Nega-\ntive Values?"=w243, "[IN] # Channel"=u8 1 ("# Channel"), "[IN] Particle Filter Setups"=w245) -> ("[OUT] Localization Settings"=w223:T8)  [unwired: 4 in]
        n87 = call "Visualize_Results_of_Filtering-1.vi"("[IN] Number of event"=i8 2, "error IN"=w239, "[IN] Localization Settings"=w223, "# Frame"="# of Frame", "[IN] Images Array"=w238) -> ("error OUT"=w234:errorcluster, "[OUT] LoG with Particles"=w235:T2, "[OUT] Binarized Image"=→"1st Filtering":T2)  [unwired: 4 in]
        "Results on 1st Movie" <- w235
        n88 = call "Localization_of_Objects-1.vi"("[IN] Detection Progress"=w230, "[IN] Number of Frames"=w228, "error IN"=w231, "[IN] Find ALL objects"="Find ALL objects", "[IN] Movie Related Values"=w224, "[IN] Localization Settings"=w223) -> ("error OUT"=w227:errorcluster, "[OUT] Movie Related Values"=w226:T12)  [unwired: 4 in]
        n89 = Merge Errors(w234, w227) -> (w253:errorcluster)
        n90 = case shown="True" "Save pics (ex)" {
          tunnel: w253 -> [w262 w264]
          tunnel: [w262 w265] -> w257
          tunnel: w235 -> [_ w263]
          frame False {
          }
          frame True {
            n91 = call "SavePics1.vi"("error IN"=w264, "default name"="Proces_Img2", "Image Dst IN"=w263) -> ("error out"=w265:errorcluster)  [unwired: 1 in]
          }
        }
      }
      event "Tracking Procedure": Value Change {
        n92 = event-data() -> ()  [unwired: 1 in, 1 out]
        n93 = control-ref of="Max angle"() -> (w290:refnum<vi>)
        n94 = control-ref of="Closing gaps"() -> (w292:refnum<vi>)
        n95 = control-ref of="Min TRK L"() -> (w289:refnum<vi>)
        n96 = control-ref of="dR min"() -> (w281:refnum<vi>)
        n97 = control-ref of="dR max"() -> (w280:refnum<vi>)
        n98 = control-ref of="% linearity"() -> (w291:refnum<vi>)
        n99 = call "Buttons_Limits(Tracking_Page)-1.vi"("[IN] dR max"=w280, "[IN] % linearity"=w291, "[IN] dR min"=w281, "[IN] Min TRK L"=w289, "error IN"=w294, "[IN] Number of Frames"=w293, "[IN] Max angle"=w290, "[IN] Closing gaps"=w292) -> ("error OUT"=w273:errorcluster)  [unwired: 3 in]
        n100 = control-ref of="Tracking progress"() -> (w282:refnum<vi>)
        n101 = Bundle("dR min"="dR min", "dR max"="dR max", "Closing gaps"="Closing gaps", "Min TRK L"="Min TRK L", "% linearity"="% linearity", "Max angle"="Max angle", "Tracking progress"=w282) -> (w275:T10)  [unwired: 1 in]
        n102 = call "Tracking_SubVI-5.vi"("[IN] Control Parameters"=w275, "error IN"=w273, "[IN] Before-After Tracks"=w274, "[IN] Movie Values"=w276) -> ("error OUT"=w269:errorcluster, "[OUT] Before-After Tracks"=w270:T13, "[OUT] Obtained Movie Values"=w272:T12, "[OUT] Number of \nRaw Displacements"=→"Raw #":i32)  [unwired: 4 in]
      }
      event "Filter Tracks": Value Change {
        n103 = event-data() -> ()  [unwired: 1 in, 1 out]
        n104 = call "Apply_Filters_to_Tracks-3.vi"("error IN"=w305, "[IN] Control Parameters"=w306, "[IN] Movie Values"=w307) -> ("error OUT"=w301:errorcluster, "[OUT] Filtered Tracks"=w302:T19, "[OUT] # Displ \nafter Filtration"=→"Saved #":i32, "[OUT] Filtered Movie Values"=w303:T12)  [unwired: 4 in, 1 out]
        n105 = control-ref of="Save pictures"() -> (w312:refnum<vi>)
        n106 = control-ref of="Delete Tracs"() -> (w311:refnum<vi>)
        n107 = control-ref of="Raw #"() -> (w315:refnum<vi>)
        n108 = control-ref of="Saved #"() -> (w314:refnum<vi>)
        n109 = control-ref of="Frame"() -> (w313:refnum<vi>)
        n110 = call "Disactivate_Frames_Until_Get_Tracking_Results-1.vi"("Delete Tracs Ref"=w311, "Save pictures Ref"=w312, "error IN"=w301, "Frame Ref"=w313, "Saved #  Ref"=w314, "Raw # Ref"=w315) -> ()  [unwired: 6 in]
        n111 = call "Calculation_Tracks_Statistics-4.vi"("error IN"=w301, "[IN] Tracks Statistics"=w299, "[IN] Filtered Tracks"=w302, "[IN] Movie Values"=w303) -> ("error OUT"=w300:errorcluster, "[OUT] Tracks Statistics"=w298:T15)  [unwired: 6 in]
      }
      event "dR min", "dR max", "Min TRK L", "Max angle", "% linearity": Value Change {
        n112 = event-data() -> ()  [unwired: 1 in, 1 out]
        n113 = property on="dR min" class="DigNum (strict)"(error in=w321) -> ("Value"=w332:dbl)  [unwired: 1 in, 2 out]
        n114 = property on="dR max" class="DigNum (strict)"(error in=w321) -> ("Value"=w326:dbl)  [unwired: 1 in, 2 out]
        n115 = property on="Max angle" class="DigNum (strict)"(error in=w321) -> ("Value"=w320:dbl)  [unwired: 1 in, 2 out]
        n116 = property on="% linearity" class="DigNum (strict)"(error in=w321) -> ("Value"=w322:i32)  [unwired: 1 in, 2 out]
        n117 = property on="Min TRK L" class="DigNum (strict)"(error in=w321) -> ("Value"=w323:i32)  [unwired: 1 in, 2 out]
        n118 = Unbundle(w333) -> ("Closing gaps"=w325:i32, "Tracking progress"=w324:refnum<vi>)  [unwired: 5 out]
        n119 = Bundle(cluster=w333, "dR min"=w332, "dR max"=w326, "Closing gaps"=w325, "Min TRK L"=w323, "% linearity"=w322, "Max angle"=w320, "Tracking progress"=w324) -> (w318:T10)
      }
      event "Show Distributions", "Bins": Value Change {
        n120 = event-data() -> ()  [unwired: 1 in, 1 out]
        n121 = call "Calculation_Statistic_Values-2.vi"("Intervals"="Bins", "[IN] Tracks Statistics"=w346) -> ("[OUT] Representation"=w344:T20)  [unwired: 3 in]
        n122 = Unbundle(w344) -> ("All Instant Vel-s"=→"All Instant Vels":T4, "mean"=→"mean Instant Vel":dbl, "standard deviation"=→"StD Instant":dbl, "All Path Vel-s"=→"All Path Vels":T4, "mean"=→"mean Path Vel":dbl, "standard deviation"=→"StD Path":dbl, "Mean Instan Vel-s"=→"Mean Instant Velocities for Each Track":T4, "Duration of tracks"=→"Duration of Tracks":T4)  [unwired: 4 out]
      }
      event "Frame", "Delete Tracs", "Save pictures": Value Change {
        w361 = i8 3 ("[IN] Number of event")
        n123 = event-data() -> ()  [unwired: 1 in, 1 out]
        n124 = Decrement(x=w378) -> (x-1=w382:u32)
        n125 = property on="Frame" class="DigNum (strict)"(error in=w363, "Maximum"=w382, "Minimum"=0.0 ("Data Entry Limits:Minimum")) -> ()  [unwired: 1 in, 2 out]
        n126 = Unbundle By Name(w384) -> ("Tracks, Coordinates"=w380:T21)
        n127 = call "Visualize_Results_of_Filtering-1.vi"("[IN] Number of event"=w361, "error IN"=w363, "[IN] Localization Settings"=w357, "# Frame"="Frame", "[IN] Images Array"=w356) -> ("error OUT"=w359:errorcluster, "[OUT] LoG with Particles"=w362:T2)  [unwired: 4 in, 1 out]
        n128 = Increment(x=w361) -> (x+1=w360:i8)
        n129 = Unbundle By Name(w380) -> ("(X,Y,dX,dY) NN filtered"=w366:dbl[][], "(X,Y,dX,dY) TH filtered"=w376:dbl[][])
        n130 = call "Visualize_Results_of_Filtering-1.vi"("[IN] Number of event"=w360, "error IN"=w359, "[IN] Localization Settings"=w357, "# Frame"="Frame", "[IN] Images Array"=w356) -> ("error OUT"=w355:errorcluster, "[OUT] LoG with Particles"=w354:T2)  [unwired: 4 in, 1 out]
        n131 = call "Paint_Tracks_on_Frame-1.vi"("Delete \nOverlay?"="Delete Tracs", "[IN] Number of event"=i8 24, "[IN] Images Array"=w356, "error IN"=w355, "# Frame"="Frame", "[IN] #1 Array (X,Y,...)"=w366, "[IN] #1 Processed Image"=w362) -> ("error OUT"=w368:errorcluster, "[OUT] #1 Overlayed Image"=w369:T2)  [unwired: 2 in]
        "1st Filtering (NN)" <- w369
        n132 = call "Paint_Tracks_on_Frame-1.vi"("Delete \nOverlay?"="Delete Tracs", "[IN] Number of event"=i8 21, "[IN] Images Array"=w356, "error IN"=w368, "# Frame"="Frame", "[IN] #1 Array (X,Y,...)"=w376, "[IN] #1 Processed Image"=w354) -> ("error OUT"=w373:errorcluster, "[OUT] #1 Overlayed Image"=w374:T2)  [unwired: 2 in]
        "1st Filtered" <- w374
        n133 = case shown="True" "Save pictures" {
          tunnel: w374 -> [_ w394]
          tunnel: w369 -> [_ w391]
          tunnel: w373 -> [w387 w393]
          tunnel: [w387 w388] -> w385
          frame False {
          }
          frame True {
            n134 = call "SavePics1.vi"("error IN"=w393, "default name"="Track_Img1", "Image Dst IN"=w394) -> ("error out"=w389:errorcluster)  [unwired: 1 in]
            n135 = call "SavePics1.vi"("error IN"=w389, "default name"="Track_Img2", "Image Dst IN"=w391) -> ("error out"=w388:errorcluster)  [unwired: 1 in]
          }
        }
      }
      event "Testing Frame", "Save pics below", "Tracks group", "Save videos \nbelow as *avi": Value Change {
        w413 = i8 5 ("[IN] Number of event")
        n136 = event-data() -> ()  [unwired: 1 in, 1 out]
        n137 = Unbundle(w423) -> ("Before Grouped Tracks"=w414:T22, "After Grouped Tracks"=w409:T22, "Current\nGroup"=w436:i32)
        n138 = Array Size(array=w414) -> (size(s)=w432:i32)
        n139 = call "Get_Info_Before-After_Tracks-1.vi"("[IN] After Tracks"=w409, "[IN] Tracks group"="Tracks group", "[IN] Before Tracks"=w414) -> ("[OUT] Maximal Frame\n(finish point all tracks)"=w430:i32, "[OUT] Min Start Pos"=w429:i32)
        n140 = Decrement(x=w432) -> (x-1=w431:i32)
        n141 = property on="Tracks group" class="DigNum (strict)"(error in=w417, "Maximum"=w431, "Minimum"=0.0 ("Data Entry Limits:Minimum")) -> (error out=w437:errorcluster)  [unwired: 1 in, 1 out]
        n142 = property on="Testing \nFrame" class="DigNum (strict)"(error in=w437, "Maximum"=w430, "Minimum"=w429) -> (error out=w435:errorcluster)  [unwired: 1 in, 1 out]
        n143 = To Unsigned Long Integer(number=w429) -> (unsigned 32bit integer=w428:u32)
        n144 = property on="Tracks \ngroup" class="DigNum (strict)"(error in=w435) -> (error out=w433:errorcluster, "Value"=w422:i32)  [unwired: 1 in, 1 out]
        n145 = in-place {
          in-place-border: w422 -> [w442]
          n146 = in-place-cluster #1(w423) -> ()  [unwired: 1 out]
          n147 = in-place-cluster #1("Current\nGroup"=w442) -> (w421:T13)
        }
        n148 = Equal?(x=w422, y=w436) -> (x = y?=w427:bool)
        n149 = case shown="True" w427 {
          tunnel: w433 -> [w445 w447]
          tunnel: w428 -> [w443 _]
          tunnel: [w444 w447] -> w416
          tunnel: [w443 w446] -> w411
          tunnel: "Testing Frame" -> [_ w446]
          frame False {
            n150 = property on="Testing \nFrame" class="DigNum (strict)"(error in=w445, "Value"=w443) -> (error out=w444:errorcluster)  [unwired: 1 in, 1 out]
          }
          frame True {
          }
        }
        n151 = call "Merge_Grouped_Tracks_Values-1.vi"("[IN] Testing Frame"=w411, "[IN] Tracks group"="Tracks group", "[IN] Grouped Tracks"=w414) -> ("[OUT] Grouped Tracks Values"=w406:T23)  [unwired: 2 in]
        n152 = call "Merge_Grouped_Tracks_Values-1.vi"("[IN] Testing Frame"=w411, "[IN] Tracks group"="Tracks group", "[IN] Grouped Tracks"=w409) -> ("[OUT] Grouped Tracks Values"=w400:T23)  [unwired: 2 in]
        n153 = call "Paint_Tracks_Before-After-4.vi"("[IN] Number of event"=w413, "[IN] Localization Settings"=w401, "[IN] Images Array"=w398, "error IN"=w416, "[IN] Grouped Tracks Values"=w406) -> ("error OUT"=w412:errorcluster, "[OUT] Image with\nDisplacements"=w415:T2)  [unwired: 5 in]
        "Connected and Grouped Tracks" <- w415
        n154 = Increment(x=w413) -> (x+1=w404:i8)
        n155 = call "Paint_Tracks_Before-After-4.vi"("[IN] Number of event"=w404, "[IN] Localization Settings"=w401, "[IN] Images Array"=w398, "error IN"=w412, "[IN] Grouped Tracks Values"=w400) -> ("error OUT"=w407:errorcluster, "[OUT] Image with\nDisplacements"=w408:T2)  [unwired: 5 in]
        "After Resolving Correspondence Problem" <- w408
        n156 = Increment(x=w404) -> (x+1=w397:i8)
        n157 = call "Save_Before-After_Tracks-4.vi"("Save movies?"="Save videos \nbelow as *avi", "[IN] Number of event"=w397, "[IN] Localization Settings"=w401, "[IN] Images Array"=w398, "error IN"=w407, "[IN] FPS"="FPS Gr", "default name"="Tracks_Before_Filt", "[IN] Grouped Tracks Values"=w406) -> ("error OUT"=w403:errorcluster)  [unwired: 3 in]
        n158 = case shown="True" "Save pics below" {
          tunnel: w415 -> [_ w451]
          tunnel: w407 -> [w448 w453]
          tunnel: [w448 w452] -> w434
          tunnel: w408 -> [_ w450]
          frame False {
          }
          frame True {
            n159 = Two Button Dialog(message="1 or 2?", 1:"After" ("F button name (\"Cancel\")"), 2:"Before" ("T button name (\"OK\")")) -> (T button?=w455:bool)
            n160 = case shown="True" w455 {
              tunnel: "Trck_ImgN" ("default name") -> [w460 w465]
              tunnel: w453 -> [w461 w464]
              tunnel: [w458 w463] -> w452
              tunnel: w451 -> [_ w462]
              tunnel: w450 -> [w459 _]
              frame False {
                n161 = call "SavePics1.vi"("error IN"=w461, "default name"=w460, "Image Dst IN"=w459) -> ("error out"=w458:errorcluster)  [unwired: 1 in]
              }
              frame True {
                n162 = call "SavePics1.vi"("error IN"=w464, "default name"=w465, "Image Dst IN"=w462) -> ("error out"=w463:errorcluster)  [unwired: 1 in]
              }
            }
          }
        }
        n163 = Increment(x=w397) -> (x+1=w396:i8)
        n164 = call "Save_Before-After_Tracks-4.vi"("Save movies?"="Save videos \nbelow as *avi", "[IN] Number of event"=w396, "[IN] Localization Settings"=w401, "[IN] Images Array"=w398, "error IN"=w403, "[IN] FPS"="FPS Gr", "default name"="Tracks_After_Filt", "[IN] Grouped Tracks Values"=w400) -> ()  [unwired: 3 in, 1 out]
      }
      event "Save movies": Value Change {
        n165 = event-data() -> ()  [unwired: 1 in, 1 out]
        n166 = Unbundle By Name(w482) -> ("Tracks, Coordinates"=w469:T21)
        n167 = Unbundle By Name(w469) -> ("(X,Y,dX,dY) TH filtered"=w478:dbl[][])
        n168 = call "Save_Tracking_Results_Movie-2.vi"("Save movies"="Save movies", "FPS"="FPS", "# codec"=4, "error IN"=w479, "AVI Refnum"=w476, "default name"="Processed_Movie1", "(X,Y,dX,dY)"=w478) -> ("error out"=w473:errorcluster)  [unwired: 4 in]
      }
      event "Save All Instant Vels", "Save Path Velocities", "Save Mean Velocities", "Save Duration of Tracks", "Save Tracks in Columns (x,y,dx,dy)": Value Change {
        n169 = event-data() -> ()  [unwired: 1 in, 1 out]
        n170 = call "Save_Various_Calculated_Vals_1.vi"("[IN] Save Tracks in Columns"="Save Tracks in Columns (x,y,dx,dy)", "[IN] Save Mean Vels for Tracks"="Save Mean Velocities", "[IN] Save Track Durations"="Save Duration of Tracks", "[IN] Save All Path Velocities"="Save Path Velocities", "error IN"=w491, "[IN] Statistics"=w493, "[IN] Save All Instant Velocities"="Save All Instant Vels", "[IN] File Path with Movie"=w490) -> ("error OUT"=w492:errorcluster)  [unwired: 3 in]
      }
      event "STOP Program": Value Change {
        n171 = event-data() -> ()  [unwired: 1 in, 1 out]
        n172 = Index Array(array=w512, index=0) -> (element=w508:T2)
        n173 = call "IMAQ AVI2 Close"("error in (no error)"=w510, "AVI Refnum"=w511) -> ("error out"=w507:errorcluster)  [unwired: 9 in]
        n174 = Request Deallocation("STOP Program") -> ()
        n175 = call "IMAQ Dispose"("All Images? (No)"=TRUE, "Image"=w508, "error in (no error)"=w507) -> ("error out"=w506:errorcluster)  [unwired: 3 in]
      }
      event Timeout {
        n176 = event-data() -> ()  [unwired: 1 in, 1 out]
      }
    }
    "error out" <- w75
    n177 = Unbundle(w75) -> ("code"=w82:i32, "source"=w81:string)  [unwired: 1 out]
    n178 = call <vilib>:"Simple Error Handler.vi"("error code (no error:0)"=w82, "error source (\" \")"=w81, "error in (no error)"=w75) -> ()  [unwired: 2 in, 5 out]
  }
  n179 = local write "Keep Nega-\ntive Values?"(TRUE ("Keep Nega-\ntive Values?")) -> ()
  n180 = local write "Closing gaps"(w17) -> ()
  n181 = local write "% linearity"(50 ("% linearity")) -> ()
  n182 = local write "Min TRK L"(w17) -> ()
  n183 = local write "dR max"(10.0 ("dR max")) -> ()
  n184 = local write "Max angle"(45.0 ("Max angle")) -> ()
  n185 = local write "dR min"(1.0 ("dR min")) -> ()
